vi "UHR-Fleezers Control (fpga) - 11.7.1UCBMeng3RG1.vi"() -> ()   [LabVIEW 2014]
doc: "UHR-Fleezers Instrument Control Code (fpga)"
uses:
  <vilib>/Platform/TimedLoop/XDataNode/timing_clust.ctl
  <vilib>/Platform/TimedLoop/XDataNode/nitl_modes.ctl
  <vilib>/Platform/TimedLoop/XDataNode/wakeup.ctl
  <vilib>/rvi/Emulation/niFpgaGetClockAttributes.vi
  <vilib>/rvi/Emulation/niFpgaSctlEmulationGetInTimedLoop.vi
  <vilib>/rvi/Emulation/niFpgaEmulationReportErrorSimple.vi
  <vilib>/rvi/Emulation/niFpgaProcessEmulError.vi
  <vilib>/rvi/DataTransferAndStorage/Container/Common/niFpgaContainerExecOnDevCompGetState.vi
  <vilib>/rvi/Emulation/niFpgaEmulationIsFPGAContextNoSignature.vi
  <vilib>/rvi/DataTransferAndStorage/Container/Common/niFpgaContainerGetUniqueNameForEmu.vi
  <vilib>/rvi/errors/nirviReportUnexpectedCaseInternalError (U32).vi
  <vilib>/rvi/Memory/Memory_Emulation/niFpgaMemoryEmulationCacheClearOnFirstRun.vi
  <vilib>/rvi/Memory/Memory_Emulation/nirvimemoryEmulationManagerCache_MakeExclusive.vi
  <vilib>/rvi/Memory/Memory_Emulation/niFpgaMemoryEmulationValidateCache.vi
  <vilib>/rvi/Memory/Memory_Emulation/nirvimemoryEmulationManagerCache_InsertValue.vi
  <vilib>/Utility/error.llb/Clear Errors.vi
  <vilib>/rvi/Memory/Memory_Emulation/nirvimemoryEmulationManagerCache_ReleaseExclusive.vi
  <vilib>/rvi/Memory/Memory_Emulation/nirvimemoryEmulationManagerCache_GetValue.vi
  <vilib>/rvi/Memory/Memory_Emulation/nirvimemoryEmulationManagerCache_SetValue.vi
  <vilib>/rvi/Emulation/niFpgaSctlEmulationResourceMgr.vi
  <vilib>/rvi/Emulation/niFpgaCriticalErrorInLSC.vi
  <vilib>/rvi/eio/common/nirviEmuTemplateMethod_errors.vi
  <vilib>/rvi/interface/RandomDataEmulation/niFpgaRandomDataHandleErrors.vi
  <vilib>/rvi/DataTransferAndStorage/Container/XNode/niFpgaContainer.xnode
  <vilib>/rvi/Memory/Memory_Emulation/niFpgaMemoryEmulationRefIn.vi
  <vilib>/eio/EIONode/EIONode.xnode
  <vilib>/eio/EIOMethodNode/EIOMethodNode.xnode
  <vilib>/rvi/interface/RandomDataEmulation/nirviRandomDataFpgaReadWriteTemplate.vi
  <vilib>/addons/control/pid/fpga.llb/XNode/niFpgaPID.xnode
  <vilib>/Platform/TimedLoop/XDataNode/XDataNode.xnode
  <vilib>/Platform/TimedLoop/XDataNode/XDNodeRunTimeDep.lvlib
panel:
  in  "Address 2":u32
  in  "Data":i64
  in  "Ready Write":bool
  in  "Tab Control":T1(tab)=enum."Force FB"
  in  "Set 3":bool
  in  "Set 2":bool=TRUE
  in  "Set 1":bool=TRUE
  in  "Trap Pos to FIFO":bool
  in  "N of AI1 Int Acq Sets":i16=2 min=1 max=3 step=1
  out "AI Late Counter":u8
  in  "ai count":u16=400
  in  "+ phase":bool
  in  "Phase count adjustment":i16
  out "Relative phase":i16
  in  "AI to FIFO":bool
  out "BD1 Frequency Out 1":u64
  out "BD1 Frequency Out 2":u64
  out "Trap Pos FIFO Timeout":u16
  out "Trap AI FIFO Timeout":u16
  in  "Trap FIFO Set Timeout":i32
  in  "Tab Control 2":T2(tab)
  in  "RD":bool
  in  "FB1 output high":i16=3000
  in  "FB1 output low":i16
  in  "D1":i16
  in  "I1":i16=5
  in  "P1":i16=10
  in  "Swap F1 and F2":bool
  in  "Cont. Scan":bool
  in  "Abort scan":bool
  in  "Cycles per step":u64
  in  "Scan BD":bool
  in  "Number of scans":u16
  in  "Scan steps":u64
  in  "Scan freq.  increment":i64
  out "Scanning":bool
  in  "Start scan":bool
  in  "OSK Bd 1":bool
  in  "Reset Bd 1":bool
  in  "PMODE":bool
  in  "Direct RF Box \nCommunication":bool
  in  "Data BD 2":u8 format="%08b"
  in  "Data BD 1":u8 format="%08b"
  in  "Address":u8 format="%02x"
  in  "Update Data":bool
  in  "FPGA Controls\n RF Box":bool
  in  "Number Interlace Cycles":u8=2 min=1 max=3
  in  "Interlace Off Parameters":u8=1 min=1 max=3
  in  "Interlace ON/OFF":bool
  out "DIO Relative phase":i16
  in  "Phase count adjustment (DIO)":i16
  in  "+ phase (DIO)":bool
  out "DIO Late Counter":u8
  in  "DIO count 1 (ticks)":u16=400
  in  "DIO count 2 (ticks)":u16=400
  in  "DIO count 3 (ticks)":u16=400
  out "AI2 Y Sum Set 2":i16
  out "AI2 Y Sum Set 1":i16
  in  "FB Setpoint Set 1":i16 min=0 step=1
  in  "FB Reset Set 1":bool
  in  "FB On/Off Set 1":bool
  in  "FB Reset Set 2":bool
  in  "FB On/Off Set 2":bool
  in  "FB Setpoint Set 2":i16 min=0 step=1
  out "Scan I":u64
  in  "Amp switch delay":u8=5
  in  "XY phase ext loop method":bool
  in  "BD 2 Amplitude 1":u16
  in  "BD 1 Amplitude 1":u16
  in  "BD 2 Frequency 1":u64
  in  "BD 1 Frequency 1":u64
  in  "BD 2 Amplitude 2":u16
  in  "BD 1 Amplitude 2":u16
  in  "BD 2 Frequency 2":u64
  in  "BD 1 Frequency 2":u64
  in  "BD 2 Amplitude 3":u16
  in  "BD 1 Amplitude 3":u16
  in  "BD 2 Frequency 3":u64
  in  "BD 1 Frequency 3":u64
  in  "BD 1 Delay (ticks)":u8
  in  "BD 2 Delay (Ticks)":u8 caption="Count(Ticks)"
  in  "Next trap write delay (ticks)":u8 caption="Count(Ticks)"
  in  "Trap 1 osc enable":bool
  in  "Trap 2 osc enable":bool
  in  "FB2 output high":fxp<+/-,16,1>=0.999969482421875
  in  "FB2 output low":fxp<+/-,16,1>=-1.0
  in  "P2":fxp<+/-,16,8> format="%.11g"
  in  "I2":fxp<+/-,16,8>=10.0 format="%.11g"
  in  "D2":fxp<+/-,16,8> format="%.11g"
  in  "Negate Diff?":bool
  in  "Diff FB Measurement?":bool
  in  "FB Trig Integrate":u32=1
  out "TTrig?":bool
  in  "TTrig Negate Pos":bool=TRUE
  out "Trap Pos FB Int Signal":fxp<+/-,24,9> format="%.18g"
  out "Trap Pos FB Int-Norm Signal":fxp<+/-,16,1> format="%.16g"
  in  "FPGA TTrig Thresh":i64
  in  "FPGA Trap Trig":bool
  out "Trap Pos FB Action":i64
  in  "Trap Pos. FB Offset Factor":i64
  in  "Trap Pos. FB Mult Factor":i64=2
  in  "Trap Pos. FB Reset":bool
  in  "Trap Pos FB Monitor T1 or T2":bool
  in  "AI1 X Scale":u16
  in  "Trap Pos FB Int Count":u16=100
  in  "Trap Pos FB Negate Action":bool
  out "AI1 X Set 2":fxp<+/-,16,1>
  out "AI1 X Set 1":fxp<+/-,16,1>
  in  "Trap Pos. FB SP":fxp<+/-,16,1>
  in  "Force feedback":bool
  out "TTrig Sig":i64
  out "TTrig Fin Thresh":i64
  in  "1D or 2D Scan?":bool
  in  "Abort scan (MCL)":bool
  in  "MCL Scan Axis":bool
  in  "Cont. Scan (MCL)":bool
  out "Scan I (MCL)":u64
  in  "Number of scans (MCL)":u16
  out "Scanning MCL":bool
  in  "Scan steps (MCL)":u64
  in  "Cycles per step (MCL)":u64
  in  "Scan freq.  increment (MCL)":i16
  in  "Start scan (MCL)":bool
  in  "AO2":i16
  in  "AO1":i16
  out "MCL Late Counter":u8
  in  "MCL count":u32=800
  out "MCL Relative Phase":i16
  in  "Phase count adjustment (MCL)":i16
  in  "+ phase (MCL)":bool
  out "APD2 int gate":bool
  out "APD3 out state":bool
  in  "APD Gate Operating Mode":u8 max=2 step=1
  in  "Invert APD Gate":bool
  in  "APD Gate OFF Count":u16=100
  in  "APD Gate ON Count":u16=300
  out "APD 1 Gate Late Counter":u8
  out "APD 1 Gate Relative Phase":i16
  in  "Phase count adjustment (APD 1 Gate)":i16
  in  "+ phase (APD 1 Gate)":bool
  out "APD 2 Counts 0":u32
  out "APD 2 Counts 1":u32
  out "APD 1 Counts 0":u32
  out "APD 1 Counts 1":u32
  out "APD1 out state":bool
  in  "APD AO scale factor":i16=1
  in  "APD to FIFO":bool
  in  "APD Acq Rate Count":u32=20000000
  out "APD Acq Late Counter":u8
  out "APD Acq Relative Phase":i16
  in  "Phase Count Adjustment (APD Acq)":i16
  in  "+ phase (APD Acq)":bool
  in  "Phase count adjustment (APD 2 Gate)":i16
  out "APD 2 Gate Late Counter":u8
  out "APD 2 Gate Relative Phase":i16
  in  "+ phase (APD 2 Gate)":bool
  out "APD2 out state":bool
  out "APD 3 Counts 0":u32
  out "APD 3 Counts 1":u32
  out "APD 3 Gate Late Counter":u8
  in  "Phase count adjustment (APD 3 Gate)":i16
  out "APD 3 Gate Relative Phase":i16
  in  "+ phase (APD 3 Gate)":bool
  out "APD1 int gate":bool
  out "APD3 int gate":bool
  in  "D3":i16
  in  "I3":i16=5
  in  "P3":i16=10
  in  "Green Filter Flipper":bool
  in  "Green FB Count":u16=1200
  out "Green Late Counter":u8
  out "Green FB Relative Phase":i16
  in  "Phase count adjustment (Green FB)":i16=10
  in  "+ phase (Green FB)":bool
  out "Green FB Sum":i16
  in  "Green int current ON count adj":u16=150
  in  "Current Out":u16=30000
  in  "Green FB On/Off":bool
  in  "Green FB Setpoint":i16=250 min=0 step=1
  in  "Green FB Reset":bool
  in  "Operating Mode 2":u8=2 max=2 step=1
  in  "Invert GI 2":bool
  in  "Green interlace OFF count 2":u16=900
  in  "Green interlace ON count 2":u16=300
  out "GI Late Counter 2":u8
  out "GI Relative phase 2":i16
  in  "Phase count adjustment (GI) 2":i16=20
  in  "+ phase (GI) 2":bool
  in  "Green interlace OFF count":u16=100
  out "GI Relative phase":i16
  in  "Phase count adjustment (GI)":i16
  in  "+ phase (GI)":bool
  in  "Green interlace ON count":u16=300
  out "GI Late Counter":u8
  in  "Invert GI":bool
  in  "Operating Mode":u8 max=2 step=1
  in  "+ phase (RI)":bool
  out "RI Relative phase":i16
  out "RI Late Counter":u8
  in  "Red interlace ON count":u16=300
  in  "Red interlace OFF count":u16=100
  in  "Invert RI":bool
  in  "Red Laser Operating Mode":u8 max=2 step=1
  in  "Phase count adjustment (RI)":i16
  out "Red FB Intensity":i16
  in  "RI Current Out":u16=30000
  in  "Red FB On/Off":bool
  in  "D4":i16
  in  "I4":i16=5
  in  "P4":i16=10
  in  "Red FB Setpoint":i16=250 min=0 step=1
  in  "Red FB Reset":bool
  in  "RI Operating Mode 2":u8=2 max=2 step=1
  in  "Invert RI 2":bool
  in  "Phase count adjustment (BI AO)":i16=20
  in  "Blue current ON count adj (AO)":u16=150
  in  "BI Current Out":i16=30000
  in  "Blue FB On/Off":bool
  in  "D5":i16
  in  "I5":i16=5
  in  "P5":i16=10
  in  "Blue FB Setpoint":i16=250 min=0 step=1
  in  "Blue FB Reset":bool
  in  "BI Operating Mode (AO)":u8=2 max=2 step=1
  in  "Invert BI (AO)":bool
  in  "Blue OFF count (AO)":u16=900
  in  "Blue ON count (AO)":u16=300
  out "BI Late Counter (AO)":u8
  out "BI Relative phase (AO)":i16
  in  "+ phase (BI AO)":bool
  in  "Phase count adjustment (BI D)":i16
  in  "Blue Laser Operating Mode (D)":u8 max=2 step=1
  in  "Invert BI (D)":bool
  in  "Blue interlace OFF count (D)":u16=100
  in  "Blue interlace ON count (D)":u16=300
  out "Blue Late Counter (D)":u8
  out "BI Relative phase (D)":i16
  in  "+ phase (BI D)":bool
  out "Blue Intensity":i16
  # "Only one of these can be on\nat a time:"
  # "Raster Scan AOD"
  # "1 (X)"
  # "2 (Y)"
  # "IR Intensity Feedback (RF BD 1)"
  # "FB Gains Set 1"
  # "FB output range 1"
  # "False is usual, True is external loop method"
  # "Parameters if using the external RF switching loop"
  # "Parameters if using the usual internal RF switching method"
  # "FB Triggering Excitation Laser"
  # "Trap Pos. FB Gains"
  # "Trap Pos. FB Range"
  # "AO1 (Y)"
  # "2D"
  # "1D"
  # "AO2 (X)"
  # "APD AO for aligning"
  # "Detection Loop"
  # "Green fluorescent laser digital gate interlacing loop"
  # "0 Forced ON\n1 Forced OFF\n2 Interlacing"
  # "Green FB Gains"
  # "Red fluorescent laser digital gate interlacing loop"
  # "Detection Loop"
  # "0 Forced ON\n1 Forced OFF\n2 Interlacing"
  # "Analog/FB Control Loop\n(Disabled)"
  # "Digital Control Loop"
  # "Blue laser intensity reading"
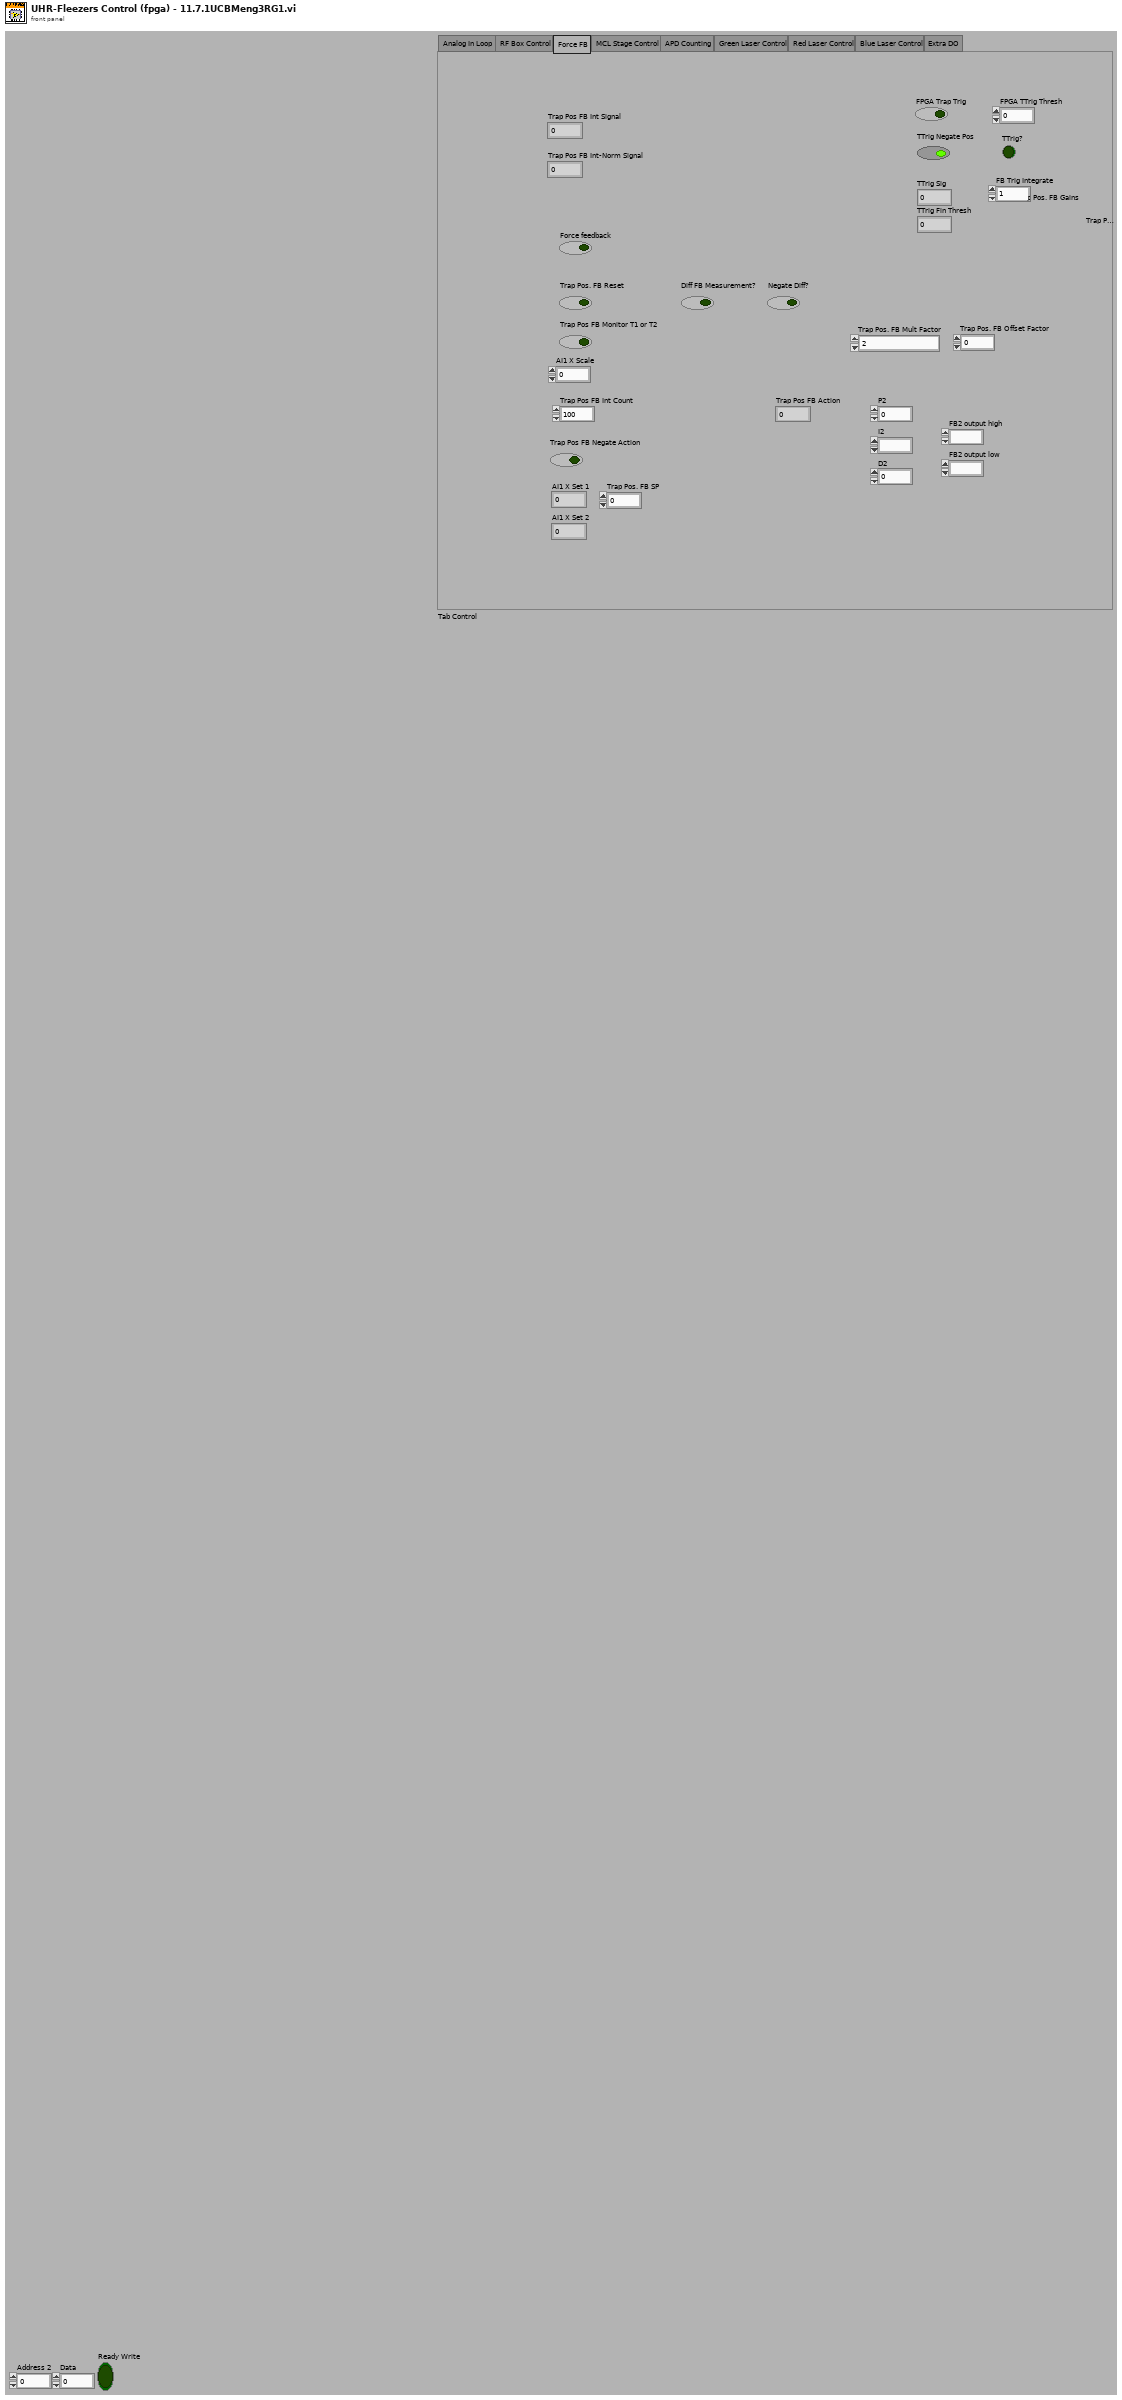
[diagram p1: front panel]
types:
  T1 = enum32{"Analog In Loop", "RF Box Control", "Force FB", "MCL Stage Control", "APD Counting", "Green Laser Control", "Red Laser Control", "Blue Laser Control", "Extra DO"}
  T2 = enum32{"Controls", "Interlacing Frequency and Amplitude Values", "Oscillate trap from memory"}
  T3 = typedef "XDNodeRunTimeDep.lvlib/timing_clust.ctl" = cluster{"Expected End [f-1]":u64, "Actual End [f-1]":u64, "Finished Late? [f-1]":bool, "Expected End [i-1]":u64, "Actual End [i-1]":u64, "Finished Late? [i-1]":bool, "Expected Start [i]":u64, "Actual Start [i]":u64, "Expected Start [f]":u64, "Actual Start [f]":u64, "Source Name":string, "Structure Name":string, "Period":i64, "Deadline":i64, "Offset":i64, "Start":i64, "Priority":i32, "Timeout":i32, "Mode":T4, "Wakeup Reason":T5, "Error":errorcluster, "Source Type":string, "Secondary Source Type":string, "Global End Time":u64, "Global Start Time":u64, "Frame Duration":u64, "Iteration Duration":u64, "Assigned CPU":i32, "I/O Scan Engine Mode":u32}
  T4 = typedef "XDNodeRunTimeDep.lvlib/nitl_modes.ctl" = enum32{"No Change", "Process missed periods, maintain original phase", "Discard missed periods, maintain original phase", "Process missed periods, ignore original phase", "Discard missed periods, ignore original phase"}
  T5 = typedef "XDNodeRunTimeDep.lvlib/wakeup.ctl" = enum32{"Normal", "Aborted", "Asynchronous wakeup", "Timing source error", "Timed loop error", "Timeout"}
  T6 = cluster{"proportional gain (Kc)":i16, "integral gain (Kc*Ts/Ti)":i16, "derivative gain (Kc*Td/Ts)":i16}
  T7 = cluster{"FB1 output high":i16, "FB1 output low":i16}
  T8 = cluster{"P2":fxp<+/-,16,8>, "I2":fxp<+/-,16,8>, "D2":fxp<+/-,16,8>}
  T9 = cluster{"FB2 output high":fxp<+/-,16,1>, "FB2 output low":fxp<+/-,16,1>}
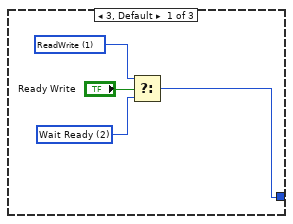
[diagram p2: hidden frame]
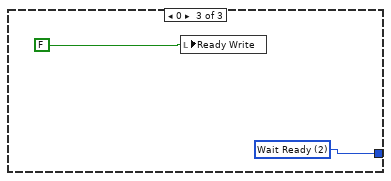
[diagram p3: hidden frame]
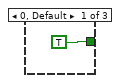
[diagram p5: hidden frame]
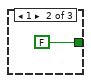
[diagram p6: hidden frame]
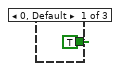
[diagram p7: hidden frame]
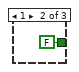
[diagram p8: hidden frame]
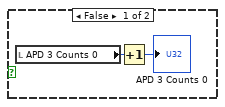
[diagram p10: hidden frame]
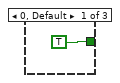
[diagram p11: hidden frame]
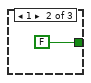
[diagram p12: hidden frame]
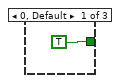
[diagram p13: hidden frame]
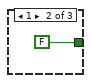
[diagram p14: hidden frame]
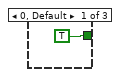
[diagram p15: hidden frame]
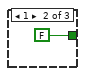
[diagram p16: hidden frame]
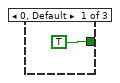
[diagram p17: hidden frame]
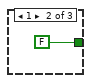
[diagram p18: hidden frame]
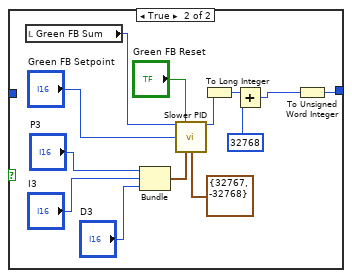
[diagram p20: hidden frame]
diagram:
  w1 = i16 2 items=["UnSet Ready", "ReadWrite", "Wait Ready"]
  w4 = u16 0
  w6 = FALSE
  w3 = FALSE
  # "timing array current index"
  # "timing array"
  # "timing counter (phase adjusted here)"
  # "late counter"
  n1 = flat-sequence "FPGA initialization to do before running any of the loops" {
    tunnel: [u16 0 ("DIO count 3 (ticks)")] -> w2
    tunnel: [w14] -> _
    frame #0 {
      w13 = FALSE ("Enable")
      # "BD 2 (Y)"
      # "BD 1 (X)"
      # "Start up expansion chassis early\nto avoid delays later"
      # "This pin controls udclk on the RF boards.\nWhen initially configuring the boards, this pin needs to be\nconfigured as a high impedance input.  Later it will be switched\nto an output."
      # "Initial setting of DIO data and \naddress to low (before reset).  \nThis needs to happen before the other\ncontrol method loops execute."
      n2 = xnode "FPGA I/O Node"("Chassis2/Mod1/AO0"=u16 0 ("Chassis2/Mod4/AO0")) -> ("Chassis2/Mod2/AI0"=w14:i16)  [unwired: 2 in, 2 out]
      n3 = xnode "FPGA I/O Method Node"("Enable"=w13) -> ()  [unwired: 1 in, 1 out]
      n4 = xnode "FPGA I/O Method Node"("Enable"=w13) -> ()  [unwired: 1 in, 1 out]
      n5 = xnode "FPGA I/O Node"("Connector1/DIO0"=FALSE, "Connector1/DIO1"=FALSE, "Connector1/DIO2"=FALSE, "Connector1/DIO3"=FALSE, "Connector1/DIO4"=FALSE, "Connector1/DIO5"=FALSE, "Connector1/DIO6"=FALSE, "Connector1/DIO7"=FALSE, "Connector1/DIO8"=FALSE, "Connector1/DIO9"=FALSE, "Connector1/DIO10"=FALSE, "Connector1/DIO11"=FALSE, "Connector1/DIO12"=FALSE, "Connector1/DIO13"=FALSE, "Connector1/DIO15"=FALSE, "Connector1/DIO20"=FALSE, "Connector1/DIO21"=FALSE, "Connector1/DIO22"=FALSE, "Connector1/DIO23"=FALSE, "Connector1/DIO24"=FALSE, "Connector1/DIO25"=FALSE, "Connector1/DIO26"=FALSE, "Connector1/DIO27"=FALSE, "Connector1/DIO14"=FALSE) -> ()  [unwired: 24 in, 24 out]
    }
  }
  n6 = local read "AO1"() -> (w11:i16)
  n7 = local read "AO2"() -> (w10:i16)
  n8 = node-c288() -> (w9:T3)  [unwired: 1 in]
  n9 = To Unsigned Long Integer(number=w2) -> (unsigned 32bit integer=w7:u32)
  n10 = timed-loop "RF box board DIO control: control bits" {
    timing: w9 -> [_]
    timing-out: [_] -> w8
    tunnel: [w43] -> _
    tunnel: w2 -> [w43]
    stop <- FALSE stop-if-true
    n11 = xnode "FPGA I/O Node"("Connector1/DIO16"="RD", "Connector1/DIO17"="PMODE", "Connector1/DIO18"="OSK Bd 1", "Connector1/DIO19"="Reset Bd 1", "Connector0/DIO3"="Green Filter Flipper") -> ()  [unwired: 5 in, 5 out]
  }
  n12 = while "RF box board direct communication loop" {
    tunnel: w2 -> [_]
    stop <- FALSE stop-if-true
    n13 = case "Whether to use direct communication method (only use one method at a time)" shown="True" "Direct RF Box \nCommunication" {
      frame False {
      }
      frame True {
        n14 = case shown="True" "Update Data" {
          frame False {
          }
          frame True {
            n15 = flat-sequence {
              frame #0 {
                n16 = First Call?() -> (First Call?: T/F=w53:bool)
                n17 = case shown="True" w53 {
                  frame False {
                  }
                  frame True {
                    # "If first time data updated, be sure to set WR high\nbefore setting data and address bits."
                    n18 = flat-sequence {
                      frame #0 {
                        n19 = xnode "FPGA I/O Node"("Connector1/DIO15"=TRUE) -> ()  [unwired: 1 in, 1 out]
                      }
                      frame #1 {
                        n20 = call "Wait"("Count(Ticks)"=u8 40 ("DO Delay 3 (Ticks)")) -> ()  [unwired: 1 out]
                      }
                    }
                  }
                }
              }
              frame #1 {
                n21 = Number To Boolean Array(number="Address") -> (Boolean array=w102:bool[])
                n22 = Number To Boolean Array(number="Data BD 1") -> (Boolean array=w103:bool[])
                n23 = Number To Boolean Array(number="Data BD 2") -> (Boolean array=w72:bool[])
                n24 = Index Array(array=w103, index=7) -> (element=w87:bool)
                n25 = Index Array(array=w103, index=6) -> (element=w86:bool)
                n26 = Index Array(array=w103, index=5) -> (element=w85:bool)
                n27 = Index Array(array=w103, index=4) -> (element=w84:bool)
                n28 = Index Array(array=w103, index=3) -> (element=w83:bool)
                n29 = Index Array(array=w103, index=2) -> (element=w82:bool)
                n30 = Index Array(array=w103, index=1) -> (element=w81:bool)
                n31 = Index Array(array=w103, index=0) -> (element=w80:bool)
                n32 = Index Array(array=w102, index=5) -> (element=w79:bool)
                n33 = Index Array(array=w102, index=4) -> (element=w78:bool)
                n34 = Index Array(array=w102, index=3) -> (element=w77:bool)
                n35 = Index Array(array=w102, index=2) -> (element=w76:bool)
                n36 = Index Array(array=w102, index=1) -> (element=w75:bool)
                n37 = Index Array(array=w102, index=0) -> (element=w74:bool)
                n38 = Index Array(array=w72, index=7) -> (element=w63:bool)
                n39 = Index Array(array=w72, index=6) -> (element=w62:bool)
                n40 = Index Array(array=w72, index=5) -> (element=w61:bool)
                n41 = Index Array(array=w72, index=4) -> (element=w60:bool)
                n42 = Index Array(array=w72, index=3) -> (element=w59:bool)
                n43 = Index Array(array=w72, index=2) -> (element=w58:bool)
                n44 = Index Array(array=w72, index=1) -> (element=w57:bool)
                n45 = Index Array(array=w72, index=0) -> (element=w56:bool)
                n46 = xnode "FPGA I/O Node"("Connector1/DIO0"=w87, "Connector1/DIO1"=w86, "Connector1/DIO2"=w85, "Connector1/DIO3"=w84, "Connector1/DIO4"=w83, "Connector1/DIO5"=w82, "Connector1/DIO6"=w81, "Connector1/DIO7"=w80, "Connector1/DIO8"=w79, "Connector1/DIO9"=w78, "Connector1/DIO10"=w77, "Connector1/DIO11"=w76, "Connector1/DIO12"=w75, "Connector1/DIO13"=w74, "Connector1/DIO20"=w63, "Connector1/DIO21"=w62, "Connector1/DIO22"=w61, "Connector1/DIO23"=w60, "Connector1/DIO24"=w59, "Connector1/DIO25"=w58, "Connector1/DIO26"=w57, "Connector1/DIO27"=w56) -> ()  [unwired: 22 in, 22 out]
              }
              frame #2 {
                # "wait and then apply write signal"
                n47 = call "Wait2"("Count(Ticks)"=u8 40 ("DO Delay 1 (Ticks)")) -> ()  [unwired: 1 out]
              }
              frame #3 {
                # "sending bit low writes data to board buffer"
                n48 = xnode "FPGA I/O Node"("Connector1/DIO15"=FALSE) -> ()  [unwired: 1 in, 1 out]
              }
              frame #4 {
                # "wait then return write signal"
                n49 = call "Wait3"("Count(Ticks)"=u8 40 ("DO Delay 2 (Ticks)")) -> ()  [unwired: 1 out]
              }
              frame #5 {
                # "sending bit high makes ready to\nwrite more data"
                n50 = xnode "FPGA I/O Node"("Connector1/DIO15"=TRUE) -> ()  [unwired: 1 in, 1 out]
              }
            }
          }
        }
      }
    }
  }
  n51 = while "RF box board DIO control: parallel communication" {
    shift-right: [w116] -> _
    shift-left: w2 -> [w115]
    shift-right: [w114] -> _
    shift-left: FALSE ("Swap F1 and F2") -> [w113]
    stop <- FALSE stop-if-true
    n52 = flat-sequence {
      tunnel: w113 -> [w120]
      tunnel: w115 -> [w118]
      tunnel: [w120] -> w112
      tunnel: [w119] -> w111
      tunnel: [w118] -> w110
      tunnel: [w126] -> w116
      tunnel: [w125] -> w114
      tunnel: w112 -> [w124]
      tunnel: w111 -> [w122]
      tunnel: w110 -> [w121]
      frame #0 {
        n53 = call "Loop Timer"("Count(Ticks)"=w118) -> ("Tick Count(Ticks)"=w119:u16)
      }
      frame #1 {
        n54 = flat-sequence {
          tunnel: ["FPGA Controls\n RF Box"] -> w123
          tunnel: w124 -> [w127]
          tunnel: [w180] -> w126
          tunnel: [w193] -> w125
          tunnel: w123 -> [w192]
          tunnel: w122 -> [w186]
          tunnel: w121 -> [w183]
          frame #0 {
            n55 = case shown="True" "FPGA Controls\n RF Box" {
              tunnel: w127 -> [_ w129]
              frame False {
              }
              frame True {
                n56 = flat-sequence {
                  tunnel: w129 -> [w139]
                  frame #0 {
                    n57 = First Call?() -> (First Call?: T/F=w130:bool)
                    n58 = case shown="True" w130 {
                      frame False {
                      }
                      frame True {
                        # "BD 2"
                        # "BD 1"
                        # "If first time data updated, be sure to set WR high and UDCLK low\nbefore setting data and address bits."
                        n59 = xnode "FPGA I/O Method Node"("Enable"=TRUE) -> ("FPGA I/O Out"=w132:refnum<k21>)  [unwired: 1 in]
                        n60 = xnode "FPGA I/O Method Node"("Enable"=TRUE) -> ("FPGA I/O Out"=w135:refnum<k21>)  [unwired: 1 in]
                        n61 = xnode "FPGA I/O Node"("Connector1/DIO15"=TRUE) -> ()  [unwired: 1 in, 1 out]
                        n62 = xnode "FPGA I/O Node"("I/O Item"=FALSE ("Connector1/DIO30"), "FPGA I/O In"=w132) -> ()  [unwired: 1 out]
                        n63 = xnode "FPGA I/O Node"("I/O Item"=FALSE ("Connector1/DIO30"), "FPGA I/O In"=w135) -> ()  [unwired: 1 out]
                      }
                    }
                  }
                  frame #1 {
                    n64 = case shown="False" FALSE {
                      tunnel: w139 -> [w141 _]
                      frame False {
                        # "Usual operation"
                        n65 = flat-sequence "BD 1 (X)" {
                          tunnel: w141 -> [w148]
                          tunnel: "Amp switch delay" -> [w149]
                          frame #0 {
                            n66 = call "Wait6"("Count(Ticks)"="BD 1 Delay (ticks)") -> ()  [unwired: 1 out]
                          }
                          frame #1 {
                            # "switch frequency"
                            n67 = xnode "FPGA I/O Node"("Connector1/DIO36"=w148) -> ()  [unwired: 1 in, 1 out]
                          }
                          frame #2 {
                            # "~5 ticks is usual"
                            n68 = call "Wait4"("Count(Ticks)"=w149) -> ()  [unwired: 1 out]
                          }
                          frame #3 {
                            # "this switches amplitude"
                            # "switch amplitude"
                            # "send udclk high"
                            n69 = xnode "FPGA I/O Node"("Connector1/DIO30"=TRUE ("Connector1/DIO15")) -> ()  [unwired: 1 in, 1 out]
                          }
                          frame #4 {
                            # "reset to be ready for next\ncycle"
                            # "send udclk low"
                            n70 = xnode "FPGA I/O Node"("Connector1/DIO30"=FALSE ("Connector1/DIO15")) -> ()  [unwired: 1 in, 1 out]
                          }
                        }
                        n71 = flat-sequence "BD 2 (Y)" {
                          tunnel: w141 -> [w143]
                          tunnel: "Amp switch delay" -> [w144]
                          frame #0 {
                            n72 = call "Wait7"("Count(Ticks)"="BD 2 Delay (Ticks)") -> ()  [unwired: 1 out]
                          }
                          frame #1 {
                            # "switch frequency"
                            n73 = xnode "FPGA I/O Node"("Connector1/DIO37"=w143) -> ()  [unwired: 1 in, 1 out]
                          }
                          frame #2 {
                            # "~5 ticks is usual"
                            n74 = call "Wait5"("Count(Ticks)"=w144) -> ()  [unwired: 1 out]
                          }
                          frame #3 {
                            # "this switches amplitude"
                            # "switch amplitude"
                            # "send udclk high"
                            n75 = xnode "FPGA I/O Node"("Connector1/DIO29"=TRUE ("Connector1/DIO15")) -> ()  [unwired: 1 in, 1 out]
                          }
                          frame #4 {
                            # "reset to be ready for next\ncycle"
                            # "send udclk low"
                            n76 = xnode "FPGA I/O Node"("Connector1/DIO29"=FALSE ("Connector1/DIO15")) -> ()  [unwired: 1 in, 1 out]
                          }
                        }
                      }
                      frame True {
                        # "Operation when you need a long delay for either X or Y to synchonize AOD light out phase (> ~100 ticks)."
                        # "Trigger the external loop by sending the boolean FSK value through a FIFO"
                      }
                    }
                  }
                }
              }
            }
          }
          frame #1 {
            # "This is the prior cycle's on time"
            # "increment timing\nindex, reset to 0 if \nend of matrix"
            # "Reset to begginning (1) when number of cycles reached."
            # "timing index"
            # "build byte stacks for writing data\n(must correspond to addresses array constant)"
            # "Timing housekeeping"
            # "Adjust phase if late\n(maintains constant phase relationship between cycles)"
            n77 = Bundle("FB1 output high"="FB1 output high", "FB1 output low"="FB1 output low") -> (w153:T7)  [unwired: 1 in]
            n78 = Bundle("P1"="P1", "I1"="I1", "D1"="D1") -> (w154:cluster{"P1":i16, "I1":i16, "D1":i16})  [unwired: 1 in]
            n79 = feedback #1(u8 0 ("t")) -> (w189:u8)
            n80 = Increment(x=w189) -> (x+1=w232:u8)
            n81 = Increment(x="Number Interlace Cycles") -> (x+1=w227:u8)
            n82 = Equal?(x=w232, y=w227) -> (x = y?=w234:bool)
            n83 = Select(t=u8 1, s=w234, f=w232) -> (s? t:f=w188:u8)
            n84 = feedback-in #1(w188) -> ()
            n85 = Increment(x=w188) -> (x+1=w229:u8)
            n86 = Equal?(x=w229, y=w227) -> (x = y?=w230:bool)
            n87 = Select(t=u8 1, s=w230, f=w229) -> (s? t:f=w226:u8)
            n88 = Select(t=w226, s="Interlace ON/OFF", f="Interlace Off Parameters") -> (s? t:f=w152:u8)
            n89 = case shown="2" w152 {
              tunnel: [w312 w468 "BD 1 Frequency 3"] -> w222
              tunnel: [w311 "BD 2 Frequency 2" "BD 2 Frequency 3"] -> w211
              tunnel: ["BD 2 Amplitude 1" "BD 2 Amplitude 2" "BD 2 Amplitude 3"] -> w168
              tunnel: [w300 w473 "BD 1 Amplitude 3"] -> w171
              tunnel: w154 -> [w274 w470 _]
              tunnel: w153 -> [w275 w469 _]
              frame 1, Default {
                w291 = fxp<+/-,24,9> 0.0 ("AI1 X Set 2")
                w284 = u16 0
                w307 = u64 0 ("f")
                # "This signal integration happens no matter what\nso that correct setpoints can be chosen before \nturning on the FB."
                # "Trap 1"
                n90 = local read "AI1 X Set 2"() -> (w287:fxp<+/-,16,1>)
                n91 = local read "AI1 X Set 1"() -> (w288:fxp<+/-,16,1>)
                n92 = local read "Scanning"() -> (w313:bool)
                n93 = Or(x=w313, y="Start scan") -> (x .or. y?=w305:bool)
                n94 = case shown="False" "Diff FB Measurement?" {
                  tunnel: w287 -> [w321 w330]
                  tunnel: w288 -> [w320 w331]
                  tunnel: [w318 w322] -> w289
                  frame False {
                    n95 = Select(t=w320, s="Trap Pos FB Monitor T1 or T2", f=w321) -> (s? t:f=w318:fxp<+/-,16,1>)
                  }
                  frame True {
                    n96 = Subtract(x=w331, y=w330) -> (x-y=w323:fxp<+/-,17,2>)
                    n97 = Not(x="Negate Diff?") -> (.not. x?=w329:bool)
                    n98 = Boolean To (0,1)(Boolean="Negate Diff?") -> (0, 1=w327:i16)
                    n99 = Boolean To (0,1)(Boolean=w329) -> (0, 1=w328:i16)
                    n100 = Negate(x=w327) -> (-x=w326:i16)
                    n101 = Add(x=w326, y=w328) -> (x+y=w324:i16)
                    n102 = Multiply(x=w324, y=w323) -> (x*y=w322:fxp<+/-,32,17>)
                  }
                }
                n103 = Not(x="Abort scan") -> (.not. x?=w303:bool)
                n104 = And(x=w303, y=w305) -> (x .and. y?=w302:bool)
                n105 = case "For raster scanning" shown="True" w302 {
                  tunnel: [u64 0 w457] -> w308
                  tunnel: "Start scan" -> [_ w442]
                  frame False {
                    n106 = local write "Scanning"(FALSE ("scanning")) -> ()
                  }
                  frame True {
                    w426 = i64 0
                    w425 = u64 0
                    # "scan incr."
                    # "freq. incr. mult."
                    # "count steps"
                    # "count number of cycles"
                    n107 = feedback #2(w425) -> (w454:u64)
                    n108 = Select(t=w425, s=w442, f=w454) -> (s? t:f=w456:u64)
                    n109 = Increment(x=w456) -> (x+1=w453:u64)
                    n110 = Greater?(x="Cycles per step", y=w453) -> (0:w435:bool)
                    n111 = Select(t=w453, s=w435, f=w425) -> (s? t:f=w452:u64)
                    n112 = feedback-in #2(w452) -> ()
                    n113 = feedback #3(w425) -> (w451:u64)
                    n114 = Select(t=w425, s=w442, f=w451) -> (s? t:f=w446:u64)
                    n115 = Increment(x=w446) -> (x+1=w450:u64)
                    n116 = Add(x="Scan steps", y="Scan steps") -> (x+y=w449:u64)
                    n117 = Select(t=w446, s=w435, f=w450) -> (s? t:f=w430:u64)
                    n118 = Greater?(x=w449, y=w430) -> (0:w429:bool)
                    n119 = Select(t=w430, s=w429, f=w425) -> (s? t:f=w447:u64)
                    n120 = feedback-in #3(w447) -> ()
                    n121 = Equal?(x="Scan steps", y=w430) -> (x = y?=w434:bool)
                    n122 = Greater?(x="Scan steps", y=w446) -> (0:w445:bool)
                    n123 = feedback #4(w426) -> (w448:i64)
                    n124 = Select(t=w426, s=w442, f=w448) -> (s? t:f=w432:i64)
                    n125 = Increment(x=w432) -> (x+1=w444:i64)
                    n126 = Decrement(x=w432) -> (x-1=w443:i64)
                    n127 = Select(t=w444, s=w445, f=w443) -> (s? t:f=w433:i64)
                    n128 = Select(t=w432, s=w434, f=w433) -> (s? t:f=w431:i64)
                    n129 = Select(t=w432, s=w435, f=w431) -> (s? t:f=w427:i64)
                    n130 = Select(t=w427, s=w429, f=w426) -> (s? t:f=w428:i64)
                    n131 = feedback-in #4(w428) -> ()
                    n132 = feedback #5(w425) -> (w441:u64)
                    n133 = Select(t=w425, s=w442, f=w441) -> (s? t:f=w437:u64)
                    n134 = Increment(x=w437) -> (x+1=w438:u64)
                    n135 = Select(t=w437, s=w429, f=w438) -> (s? t:f=w436:u64)
                    n136 = Greater?(x="Number of scans", y=w436) -> (0:w422:bool)
                    n137 = Multiply(x="Scan freq.  increment", y=w432) -> (x*y=w457:i64)
                    n138 = Select(t=TRUE, s="Cont. Scan", f=w422) -> (s? t:f=w421:bool)
                    "Scanning" <- w421
                    n139 = Select(t=w436, s=w421, f=w425) -> (s? t:f=w439:u64)
                    n140 = feedback-in #5(w439) -> ()
                    n141 = Increment(x=w436) -> (x+1=→"Scan I":u64)
                  }
                }
                n142 = feedback #6(w284) -> (w283:u16)
                n143 = Increment(x=w283) -> (x+1=w285:u16)
                n144 = Greater Or Equal?(x=w285, y="Trap Pos FB Int Count") -> (x >= y?=w276:bool)
                n145 = Select(t=w284, s=w276, f=w285) -> (s? t:f=w286:u16)
                n146 = feedback-in #6(w286) -> ()
                n147 = feedback #7(w291) -> (w290:fxp<+/-,24,9>)
                n148 = Add(x=w289, y=w290) -> (x+y=w282:fxp<+/-,24,9>)
                n149 = case "For intensity feedback" shown="True" "FB On/Off Set 1" {
                  tunnel: "BD 1 Amplitude 1" -> [w459 _]
                  tunnel: [w459 w463] -> w300
                  tunnel: w275 -> [_ w460]
                  tunnel: w274 -> [_ w461]
                  frame False {
                  }
                  frame True {
                    n150 = local read "AI2 Y Sum Set 1"() -> (w464:i16)
                    n151 = call "Slower PID.vi"("process variable"=w464, "reset?"="FB Reset Set 1", "setpoint"="FB Setpoint Set 1", "PID gains (x 2^8)"=w461, "output range"=w460) -> ("output"=w465:i16)  [unwired: 10 out]
                    n152 = To Unsigned Word Integer(number=w465) -> (unsigned 16bit integer=w463:u16)
                  }
                }
                n153 = Select(t=w291, s=w276, f=w282) -> (s? t:f=w294:fxp<+/-,24,9>)
                n154 = feedback-in #7(w294) -> ()
                n155 = Divide(x=w282, y="Trap Pos FB Int Count") -> (x/y=w277:fxp<+/-,16,1>)
                n156 = feedback #8(fxp<+/-,24,9> 0.0 ("AI1 X Set 2")) -> (w295:fxp<+/-,24,9>)
                n157 = Select(t=w282, s=w276, f=w295) -> (s? t:f=w296:fxp<+/-,24,9>)
                "Trap Pos FB Int Signal" <- w296
                n158 = feedback-in #8(w296) -> ()
                n159 = feedback #9(fxp<+/-,16,1> 0.0 ("Trap Pos FB Int-Norm Signal")) -> (w279:fxp<+/-,16,1>)
                n160 = Select(t=w277, s=w276, f=w279) -> (s? t:f=w278:fxp<+/-,16,1>)
                "Trap Pos FB Int-Norm Signal" <- w278
                n161 = feedback-in #9(w278) -> ()
                n162 = case "For position feedback" shown="True" "Force feedback" {
                  tunnel: [i64 0 w337] -> w297
                  tunnel: w277 -> [_ w334]
                  tunnel: w276 -> [_ w333]
                  frame False {
                  }
                  frame True {
                    n163 = feedback #10(i64 0) -> (w336:i64)
                    n164 = case shown="True" w333 {
                      tunnel: [w338 w352] -> w337
                      tunnel: w336 -> [w338 _]
                      tunnel: w334 -> [_ w346]
                      frame False {
                      }
                      frame True {
                        w356 = u32 0
                        n165 = Bundle("P2"="P2", "I2"="I2", "D2"="D2") -> (w342:T8)  [unwired: 1 in]
                        n166 = Bundle("FB2 output high"="FB2 output high", "FB2 output low"="FB2 output low") -> (w339:T9)  [unwired: 1 in]
                        n167 = xnode ("PID")("process variable"=w346, "reset?"="Trap Pos. FB Reset", "setpoint"="Trap Pos. FB SP", "PID gains"=w342, "output range"=w339) -> ("output"=w368:fxp<+/-,16,1>)
                        n168 = Negate(x=w368) -> (-x=w367:fxp<+/-,17,2>)
                        n169 = Select(t=w367, s="Trap Pos FB Negate Action", f=w368) -> (s? t:f=w364:fxp<+/-,17,2>)
                        n170 = Scale By Power Of 2(n=u32 15, x=u32 1) -> (x*2^n=w361:u32)
                        n171 = Multiply(x=w364, y=w361) -> (x*y=w360:fxp<+/-,17,17>)
                        n172 = To Quad Integer(1:w360) -> (0:w372:i64)
                        "Trap Pos FB Action" <- w372
                        n173 = Multiply(x=w372, y="Trap Pos. FB Mult Factor") -> (x*y=w370:i64)
                        n174 = Add(x=w370, y="Trap Pos. FB Offset Factor") -> (x+y=w352:i64)
                        n175 = feedback #11() -> (w353:i64)  [unwired: 1 in]
                        n176 = Add(x=w352, y=w353) -> (x+y=w350:i64)
                        n177 = feedback #12(w356) -> (w358:u32)
                        n178 = Increment(x=w358) -> (x+1=w347:u32)
                        n179 = Greater Or Equal?(x=w347, y="FB Trig Integrate") -> (x >= y?=w348:bool)
                        n180 = Select(t=i64 0, s=w348, f=w350) -> (s? t:f=w354:i64)
                        n181 = feedback-in #11(w354) -> ()
                        n182 = Select(t=w356, s=w348, f=w347) -> (s? t:f=w357:u32)
                        n183 = feedback-in #12(w357) -> ()
                        n184 = And(x=w348, y="FPGA Trap Trig") -> (x .and. y?=w355:bool)
                        n185 = case "Trap FB trigger excitation laser ON" shown="True" w355 {
                          tunnel: w350 -> [_ w376]
                          tunnel: w347 -> [_ w374]
                          frame False {
                          }
                          frame True {
                            n186 = Not(x="TTrig Negate Pos") -> (.not. x?=w383:bool)
                            n187 = Boolean To (0,1)(Boolean="TTrig Negate Pos") -> (0, 1=w381:i16)
                            n188 = Boolean To (0,1)(Boolean=w383) -> (0, 1=w382:i16)
                            n189 = Negate(x=w381) -> (-x=w380:i16)
                            n190 = Add(x=w380, y=w382) -> (x+y=w379:i16)
                            n191 = Multiply(x=w379, y=w376) -> (x*y=w378:i64)
                            "TTrig Sig" <- w378
                            n192 = Multiply(x="FPGA TTrig Thresh", y=w374) -> (x*y=w375:i64)
                            "TTrig Fin Thresh" <- w375
                            n193 = Greater Or Equal?(x=w378, y=w375) -> (x >= y?=w377:bool)
                            n194 = case shown="True" w377 {
                              frame False {
                              }
                              frame True {
                                w386 = TRUE ("Green FB On/Off")
                                w388 = u8 2 ("Operating Mode")
                                n195 = local write "Operating Mode 2"(w388) -> ()
                                n196 = local write "Operating Mode"(w388) -> ()
                                n197 = local write "Green FB On/Off"(w386) -> ()
                                n198 = local write "FPGA Trap Trig"(FALSE ("FPGA Trap Trig")) -> ()
                                "TTrig?" <- w386
                              }
                            }
                          }
                        }
                      }
                    }
                    n199 = feedback-in #10(w337) -> ()
                  }
                }
                n200 = Select(t=w307, s="Scan BD", f=w308) -> (s? t:f=w306:u64)
                n201 = Select(t=w308, s="Scan BD", f=w307) -> (s? t:f=w309:u64)
                n202 = Add(x=w306, y="BD 2 Frequency 1") -> (x+y=w311:u64)
                n203 = Compound Arithmetic op=ADD(i64 0 ("f"), "BD 1 Frequency 1", w297, w309) -> (w312:u64)
                "BD1 Frequency Out 1" <- w312
              }
              frame 2 {
                # "Trap 2"
                n204 = case shown="True" "FB On/Off Set 2" {
                  tunnel: [w477 w480] -> w473
                  tunnel: "BD 1 Amplitude 2" -> [w477 _]
                  tunnel: w470 -> [_ w479]
                  tunnel: w469 -> [_ w478]
                  frame False {
                  }
                  frame True {
                    n205 = local read "AI2 Y Sum Set 2"() -> (w483:i16)
                    n206 = call "Slower PID.vi"("process variable"=w483, "reset?"="FB Reset Set 2", "setpoint"="FB Setpoint Set 2", "PID gains (x 2^8)"=w479, "output range"=w478) -> ("output"=w481:i16)  [unwired: 10 out]
                    n207 = To Unsigned Word Integer(number=w481) -> (unsigned 16bit integer=w480:u16)
                  }
                }
                n208 = Add(x="BD 1 Frequency 2", y=i64 0 ("f")) -> (x+y=w468:u64)
                "BD1 Frequency Out 2" <- w468
              }
              frame 3 {
                # "Fluorescence period"
              }
            }
            n209 = feedback-in #13(w186) -> ()
            n210 = feedback #13(w186) -> (w185:u16)
            n211 = Select(t=w188, s="Interlace ON/OFF", f="Interlace Off Parameters") -> (s? t:f=w225:u8)
            n212 = Subtract(x=w186, y=w185) -> (x-y=w184:u16)
            n213 = Subtract "The error"(x=w184, y=w183) -> (x-y=w161:u16)
            n214 = case shown="1, Default" w225 {
              tunnel: ["DIO count 1 (ticks)" "DIO count 2 (ticks)" "DIO count 3 (ticks)"] -> w182
              frame 1, Default {
              }
              frame 2 {
              }
              frame 3 {
              }
            }
            n215 = Number To Boolean Array(number=w161) -> (Boolean array=w162:bool[])
            n216 = Or Array Elements(Boolean array=w162) -> (logical OR=w160:bool)
            n217 = Boolean To (0,1)(Boolean=w160) -> (0, 1=w167:i16)
            n218 = To Unsigned Byte Integer(number=w167) -> (unsigned 8bit integer=w164:u8)
            n219 = feedback #14(u8 0) -> (w165:u8)
            n220 = Add(x=w164, y=w165) -> (x+y=w163:u8)
            "DIO Late Counter" <- w163
            n221 = feedback-in #14(w163) -> ()
            n222 = Subtract(x=w182, y=w161) -> (x-y=w181:u16)
            n223 = Split Number(x=w222) -> (hi(x)=w221:u32, lo(x)=w220:u32)
            n224 = Split Number(x=w211) -> (hi(x)=w216:u32, lo(x)=w215:u32)
            n225 = Boolean To (0,1)(Boolean="+ phase (DIO)") -> (0, 1=w178:i16)
            n226 = Split Number(x=w221) -> (lo(x)=w219:u16)  [unwired: 1 out]
            n227 = Split Number(x=w220) -> (hi(x)=w218:u16, lo(x)=w217:u16)
            n228 = Split Number(x=w216) -> (lo(x)=w214:u16)  [unwired: 1 out]
            n229 = Split Number(x=w215) -> (hi(x)=w213:u16, lo(x)=w212:u16)
            n230 = Split Number(x=w171) -> (hi(x)=w173:u8, lo(x)=w172:u8)
            n231 = Split Number(x=w168) -> (hi(x)=w170:u8, lo(x)=w169:u8)
            n232 = Split Number(x=w219) -> (hi(x)=w210:u8, lo(x)=w209:u8)
            n233 = Split Number(x=w218) -> (hi(x)=w208:u8, lo(x)=w207:u8)
            n234 = Split Number(x=w214) -> (hi(x)=w203:u8, lo(x)=w202:u8)
            n235 = Split Number(x=w217) -> (hi(x)=w206:u8, lo(x)=w205:u8)
            n236 = Split Number(x=w213) -> (hi(x)=w201:u8, lo(x)=w200:u8)
            n237 = Split Number(x=w212) -> (hi(x)=w199:u8, lo(x)=w198:u8)
            n238 = Multiply(x=w178, y="Phase count adjustment (DIO)") -> (x*y=w174:i16)
            n239 = feedback #15(i16 0) -> (w176:i16)
            n240 = Subtract(x=w176, y=w174) -> (x-y=w175:i16)
            "DIO Relative phase" <- w175
            n241 = feedback-in #15(w175) -> ()
            n242 = Add(x=w181, y=w174) -> (x+y=w180:u16)
            n243 = Build Array "BD 1 A Stack"(w173, w172) -> (w195:u8[])
            n244 = Build Array "BD 2 A Stack"(w170, w169) -> (w194:u8[])
            n245 = Build Array "BD 1 nu Stack"(w210, w209, w208, w207, w206, w205) -> (w204:u8[])
            n246 = Build Array "BD 2 nu Stack"(w203, w202, w201, w200, w199, w198) -> (w197:u8[])
            n247 = case shown="2" w152 {
              tunnel: [w265 w268] -> w193
              tunnel: [u8 10 u8 4] -> w196
              tunnel: "Swap F1 and F2" -> [w266 w268]
              frame 2 {
                # "F2"
                n248 = Not(x=w266) -> (.not. x?=w265:bool)
              }
              frame 1, Default {
                # "low chooses F1"
                # "F1"
              }
            }
            n249 = case "If FPGA is controlling (toggling) RF synth" shown="True" w192 {
              tunnel: w204 -> [_ w241]
              tunnel: w197 -> [_ w240]
              tunnel: w196 -> [_ w239]
              tunnel: w195 -> [_ w238]
              tunnel: w194 -> [_ w237]
              frame False {
              }
              frame True {
                # "Write next amp.\n(wait until beginning of next loop iteration to update)"
                n250 = flat-sequence "Update the next F1 and F2 frequency value (the actual frequency won't change until FSK is switched).\nThen load the next amplitude value into buffer, but don't update it until the next cycle." {
                  tunnel: w240 -> [w243]
                  tunnel: w241 -> [w244]
                  tunnel: [w244] -> w236
                  tunnel: [w243] -> w235
                  tunnel: w239 -> [w245]
                  tunnel: w236 -> [w247]
                  tunnel: w235 -> [w246]
                  tunnel: w238 -> [w258]
                  tunnel: w237 -> [w257]
                  frame #0 {
                    # "To possibly send\nthese writes to very\nend of loop (for x and\ny phase adjust)"
                    n251 = call "Wait8"("Count(Ticks)"="Next trap write delay (ticks)") -> ()  [unwired: 1 out]
                  }
                  frame #1 {
                    n252 = for {
                      tunnel: w247 -> [w253] mode=indexing
                      tunnel: w246 -> [w252] mode=indexing
                      tunnel: w245 -> [w250]
                      i -> [w251]
                      # "Write next freq."
                      n253 = To Unsigned Byte Integer(number=w251) -> (unsigned 8bit integer=w248:u8)
                      n254 = Add(x=w250, y=w248) -> (x+y=w249:u8)
                      n255 = call "write to RF synth bd.vi"("Address Byte"=w249, "BD 2 Byte"=w252, "BD 1 Byte"=w253) -> ()
                    }
                  }
                  frame #2 {
                    w254 = TRUE ("Connector1/DIO15")
                    # "send udclk high\n(BD 1 and 2)"
                    n256 = xnode "FPGA I/O Node"("Connector1/DIO30"=w254, "Connector1/DIO29"=w254) -> ()  [unwired: 2 in, 2 out]
                  }
                  frame #3 {
                    w255 = FALSE ("Connector1/DIO15")
                    n257 = xnode "FPGA I/O Node"("Connector1/DIO30"=w255, "Connector1/DIO29"=w255) -> ()  [unwired: 2 in, 2 out]
                  }
                  frame #4 {
                    n258 = for {
                      tunnel: w258 -> [w264] mode=indexing
                      tunnel: w257 -> [w263] mode=indexing
                      tunnel: u8 33 -> [w261]
                      i -> [w262]
                      n259 = To Unsigned Byte Integer(number=w262) -> (unsigned 8bit integer=w259:u8)
                      n260 = Add(x=w261, y=w259) -> (x+y=w260:u8)
                      n261 = call "write to RF synth bd.vi"("Address Byte"=w260, "BD 2 Byte"=w263, "BD 1 Byte"=w264) -> ()
                    }
                  }
                }
              }
            }
          }
        }
      }
    }
  }
  n262 = while "APD 1 Counter" {
    tunnel: w2 -> [_]
    stop <- FALSE stop-if-true
    n263 = flat-sequence {
      frame #0 {
        n264 = xnode "FPGA I/O Method Node"("FPGA I/O In"=refnum<k21> "Connector0/DIO0" ("APD 1 DO"), "Timeout"=-1) -> ()  [unwired: 2 out]
      }
      frame #1 {
        n265 = local read "APD1 int gate"() -> (w492:bool)
        n266 = case shown="True" w492 {
          frame False {
          }
          frame True {
            n267 = local read "APD1 out state"() -> (w493:bool)
            n268 = case shown="True" w493 {
              frame False {
                n269 = local read "APD 1 Counts 0"() -> (w495:u32)
                n270 = Increment(x=w495) -> (x+1=→"APD 1 Counts 0":u32)
              }
              frame True {
                n271 = local read "APD 1 Counts 1"() -> (w497:u32)
                n272 = Increment(x=w497) -> (x+1=→"APD 1 Counts 1":u32)
              }
            }
          }
        }
      }
    }
  }
  n273 = while "Handshake memory transfer for trap oscillation sin wave data" {
    shift-right: [w499] -> _
    shift-left: w1 -> [w500]
    stop <- FALSE stop-if-true
    # "Write"
    n274 = case shown="1" w500 {
      tunnel: [w503 w508 w509] -> w499
      frame 3, Default {
        w501 = i16 2 items=["UnSet Ready", "ReadWrite", "Wait Ready"]
        w502 = i16 1 items=["UnSet Ready", "ReadWrite", "Wait Ready"]
        n275 = Select(t=w502, s="Ready Write", f=w501) -> (s? t:f=w503:i16)
      }
      frame 1 {
        w508 = i16 0 items=["UnSet Ready", "ReadWrite", "Wait Ready"]
        n276 = xnode ("Memory Write")("Address"="Address 2", "Data"="Data", "Memory In"=refnum<k21> "Trap osc memory") -> ()  [unwired: 1 out]
      }
      frame 0 {
        w509 = i16 2 items=["UnSet Ready", "ReadWrite", "Wait Ready"]
        n277 = local write "Ready Write"(FALSE ("Ready Read")) -> ()
      }
    }
  }
  n278 = while "APD 2 Counter" {
    tunnel: w2 -> [_]
    stop <- FALSE stop-if-true
    n279 = flat-sequence {
      frame #0 {
        n280 = xnode "FPGA I/O Method Node"("FPGA I/O In"=refnum<k21> "Connector0/DIO1" ("APD 2 DO"), "Timeout"=-1) -> ()  [unwired: 2 out]
      }
      frame #1 {
        n281 = local read "APD2 int gate"() -> (w514:bool)
        n282 = case shown="True" w514 {
          frame False {
          }
          frame True {
            n283 = local read "APD2 out state"() -> (w515:bool)
            n284 = case shown="False" w515 {
              frame False {
                n285 = local read "APD 2 Counts 0"() -> (w517:u32)
                n286 = Increment(x=w517) -> (x+1=→"APD 2 Counts 0":u32)
              }
              frame True {
                n287 = local read "APD 2 Counts 1"() -> (w519:u32)
                n288 = Increment(x=w519) -> (x+1=→"APD 2 Counts 1":u32)
              }
            }
          }
        }
      }
    }
  }
  n289 = while "APD 2 Gating" {
    shift-right: [w523] -> _
    shift-left: w2 -> [w528]
    shift-right: [w522] -> _
    shift-left: w6 -> [w520]
    stop <- FALSE stop-if-true
    n290 = flat-sequence {
      tunnel: w528 -> [w531]
      tunnel: [w532] -> w526
      tunnel: [w531] -> w524
      tunnel: [w530] -> w521
      tunnel: w520 -> [w530]
      tunnel: [w535] -> w527
      tunnel: w526 -> [w535]
      tunnel: [w534] -> w525
      tunnel: w524 -> [w534]
      tunnel: w521 -> [w533]
      tunnel: [w557] -> w523
      tunnel: w527 -> [w567]
      tunnel: w525 -> [w565]
      tunnel: [w536] -> w522
      frame #0 {
        n291 = call "Loop Timer8"("Count(Ticks)"=w531) -> ("Tick Count(Ticks)"=w532:u16)
      }
      frame #1 {
        # "Signal maybe then sent through \na transistor before APD"
        n292 = xnode "FPGA I/O Node"("Connector0/DIO8"=w533, "Connector0/DIO9"=w533, "Connector0/DIO10"=w533, "Connector0/DIO11"=w533) -> ()  [unwired: 4 in, 4 out]
        "APD2 int gate" <- w533
      }
      frame #2 {
        n293 = local read "APD Gate ON Count"() -> (w550:u16)
        n294 = local read "APD Gate OFF Count"() -> (w549:u16)
        n295 = feedback #16(TRUE) -> (w562:bool)
        n296 = feedback-in #17(w567) -> ()
        n297 = feedback #17(w567) -> (w551:u16)
        n298 = Not(x=w562) -> (.not. x?=w560:bool)
        n299 = feedback-in #16(w560) -> ()
        n300 = Subtract(x=w567, y=w551) -> (x-y=w566:u16)
        n301 = Select(t=w550, s=w560, f=w549) -> (s? t:f=w564:u16)
        n302 = Subtract(x=w566, y=w565) -> (x-y=w542:u16)
        n303 = Subtract(x=w564, y=w542) -> (x-y=w556:u16)
        n304 = Number To Boolean Array(number=w542) -> (Boolean array=w541:bool[])
        n305 = Or Array Elements(Boolean array=w541) -> (logical OR=w540:bool)
        n306 = Boolean To (0,1)(Boolean="+ phase (APD 2 Gate)") -> (0, 1=w554:i16)
        n307 = Multiply(x=w554, y="Phase count adjustment (APD 2 Gate)") -> (x*y=w552:i16)
        n308 = Boolean To (0,1)(Boolean=w540) -> (0, 1=w547:i16)
        n309 = Add(x=w556, y=w552) -> (x+y=w557:u16)
        n310 = To Unsigned Byte Integer(number=w547) -> (unsigned 8bit integer=w544:u8)
        n311 = feedback #18(i16 0) -> (w559:i16)
        n312 = Subtract(x=w559, y=w552) -> (x-y=w558:i16)
        "APD 2 Gate Relative Phase" <- w558
        n313 = feedback-in #18(w558) -> ()
        n314 = feedback #19(u8 0) -> (w545:u8)
        n315 = Add(x=w544, y=w545) -> (x+y=w543:u8)
        "APD 2 Gate Late Counter" <- w543
        n316 = feedback-in #19(w543) -> ()
        n317 = local read "APD Gate Operating Mode"() -> (w548:u8)
        n318 = case shown="2" w548 {
          tunnel: [TRUE FALSE w570] -> w537
          tunnel: w562 -> [_ _ w570]
          frame 0, Default {
          }
          frame 1 {
          }
          frame 2 {
          }
        }
        n319 = local read "Invert APD Gate"() -> (w539:bool)
        n320 = Not(x=w537) -> (.not. x?=w538:bool)
        n321 = Select(t=w538, s=w539, f=w537) -> (s? t:f=w536:bool)
      }
    }
  }
  n322 = while "532 nm green fluorescent laser interlacing (DO to IA 532 nm AOM ME amp)." {
    shift-right: [w574] -> _
    shift-left: w2 -> [w579]
    shift-right: [w573] -> _
    shift-left: w3 -> [w571]
    stop <- FALSE stop-if-true
    n323 = flat-sequence {
      tunnel: w579 -> [w582]
      tunnel: [w583] -> w577
      tunnel: [w582] -> w575
      tunnel: [w581] -> w572
      tunnel: w571 -> [w581]
      tunnel: [w586] -> w578
      tunnel: w577 -> [w586]
      tunnel: [w585] -> w576
      tunnel: w575 -> [w585]
      tunnel: w572 -> [w584]
      tunnel: [w595] -> w574
      tunnel: w578 -> [w615]
      tunnel: w576 -> [w612]
      tunnel: [w604] -> w573
      frame #0 {
        n324 = call "Loop Timer4"("Count(Ticks)"=w582) -> ("Tick Count(Ticks)"=w583:u16)
      }
      frame #1 {
        n325 = xnode "FPGA I/O Node"("Connector1/DIO34"=w584, "Connector1/DIO38"=w584, "Connector1/DIO39"=w584) -> ()  [unwired: 3 in, 3 out]
      }
      frame #2 {
        n326 = feedback-in #20(w615) -> ()
        n327 = feedback #20(w615) -> (w614:u16)
        n328 = Subtract(x=w615, y=w614) -> (x-y=w613:u16)
        n329 = Subtract(x=w613, y=w612) -> (x-y=w588:u16)
        n330 = Number To Boolean Array(number=w588) -> (Boolean array=w589:bool[])
        n331 = Or Array Elements(Boolean array=w589) -> (logical OR=w587:bool)
        n332 = Boolean To (0,1)(Boolean="+ phase (GI)") -> (0, 1=w600:i16)
        n333 = Multiply(x=w600, y="Phase count adjustment (GI)") -> (x*y=w597:i16)
        n334 = Boolean To (0,1)(Boolean=w587) -> (0, 1=w594:i16)
        n335 = To Unsigned Byte Integer(number=w594) -> (unsigned 8bit integer=w591:u8)
        n336 = feedback #21(i16 0) -> (w598:i16)
        n337 = feedback #22(u8 0) -> (w592:u8)
        n338 = Add(x=w591, y=w592) -> (x+y=w590:u8)
        "GI Late Counter" <- w590
        n339 = feedback-in #22(w590) -> ()
        n340 = Subtract(x=w598, y=w597) -> (x-y=w596:i16)
        "GI Relative phase" <- w596
        n341 = feedback-in #21(w596) -> ()
        n342 = feedback #23(TRUE) -> (w607:bool)
        n343 = case shown="2" "Operating Mode" {
          tunnel: [TRUE FALSE w621] -> w604
          tunnel: w607 -> [_ _ w618]
          frame 0, Default {
          }
          frame 1 {
          }
          frame 2 {
            n344 = Not(x=w618) -> (.not. x?=w620:bool)
            n345 = Select(t=w620, s="Invert GI", f=w618) -> (s? t:f=w621:bool)
          }
        }
        n346 = Not(x=w607) -> (.not. x?=w603:bool)
        n347 = Select(t="Green interlace ON count", s=w603, f="Green interlace OFF count") -> (s? t:f=w609:u16)
        n348 = Subtract(x=w609, y=w588) -> (x-y=w601:u16)
        n349 = Add(x=w601, y=w597) -> (x+y=w595:u16)
        n350 = feedback-in #23(w603) -> ()
      }
    }
  }
  n351 = while "Green and red fluorescent laser interlacing (Current AO to IA 532 nm AOM ME amp)." {
    shift-right: [w630] -> _
    shift-left: w2 -> [w633]
    shift-right: [w627] -> _
    shift-left: w4 -> [w625]
    shift-right: [w624] -> _
    shift-left: w4 -> [w623]
    stop <- FALSE stop-if-true
    n352 = flat-sequence {
      tunnel: w633 -> [w637]
      tunnel: [w638] -> w632
      tunnel: [w637] -> w631
      tunnel: [w636] -> w626
      tunnel: w625 -> [w636]
      tunnel: w623 -> [w635]
      tunnel: [w635] -> w622
      tunnel: [w642] -> w629
      tunnel: w632 -> [w642]
      tunnel: [w641] -> w628
      tunnel: w631 -> [w641]
      tunnel: w626 -> [w640]
      tunnel: w622 -> [w639]
      tunnel: [w663] -> w630
      tunnel: [w679] -> w627
      tunnel: w629 -> [w690]
      tunnel: w628 -> [w687]
      tunnel: [w647] -> w624
      frame #0 {
        n353 = call "Loop Timer10"("Count(Ticks)"=w637) -> ("Tick Count(Ticks)"=w638:u16)
      }
      frame #1 {
        n354 = xnode "FPGA I/O Node"("Chassis2/Mod1/AO0"=w640, "Chassis2/Mod1/AO1"=w639) -> ()  [unwired: 2 in, 2 out]
      }
      frame #2 {
        # "Design note:\n\nThese two laser controls are in the same loop\nbecause the expansion current AI cannot separately\ntime the outputs fast enough for us.  Apparently\nit is because of communication time between the\nexpansion card and the fpga.\n\nSo the two analog control signals have the same timing\nand profile, but independent amplitudes to independently\ncontrol the intensity and feedback for each laser."
        n355 = feedback #24(TRUE) -> (w643:bool)
        n356 = Not(x=w643) -> (.not. x?=w644:bool)
        n357 = feedback-in #24(w644) -> ()
        n358 = Subtract(x="Green interlace OFF count 2", y="Green int current ON count adj") -> (x-y=w672:u16)
        n359 = feedback-in #25(w690) -> ()
        n360 = feedback #25(w690) -> (w689:u16)
        n361 = Add(x="Green int current ON count adj", y="Green interlace ON count 2") -> (x+y=w673:u16)
        n362 = Subtract(x=w690, y=w689) -> (x-y=w688:u16)
        n363 = Select(t=w673, s=w644, f=w672) -> (s? t:f=w684:u16)
        n364 = Subtract(x=w688, y=w687) -> (x-y=w656:u16)
        n365 = case shown="2" "RI Operating Mode 2" {
          tunnel: [TRUE FALSE w696] -> w645
          tunnel: w643 -> [_ _ w693]
          frame 0, Default {
          }
          frame 1 {
          }
          frame 2 {
            n366 = Not(x=w693) -> (.not. x?=w695:bool)
            n367 = Select(t=w695, s="Invert RI 2", f=w693) -> (s? t:f=w696:bool)
          }
        }
        n368 = Subtract(x=w684, y=w656) -> (x-y=w667:u16)
        n369 = case shown="0, Default" "Operating Mode 2" {
          tunnel: [TRUE FALSE w730] -> w648
          tunnel: w643 -> [_ _ w727]
          frame 0, Default {
          }
          frame 1 {
          }
          frame 2 {
            n370 = Not(x=w727) -> (.not. x?=w729:bool)
            n371 = Select(t=w729, s="Invert GI 2", f=w727) -> (s? t:f=w730:bool)
          }
        }
        n372 = Number To Boolean Array(number=w656) -> (Boolean array=w657:bool[])
        n373 = Boolean To (0,1)(Boolean="+ phase (GI) 2") -> (0, 1=w669:i16)
        n374 = Or Array Elements(Boolean array=w657) -> (logical OR=w655:bool)
        n375 = Boolean To (0,1)(Boolean=w655) -> (0, 1=w662:i16)
        n376 = Multiply(x=w669, y="Phase count adjustment (GI) 2") -> (x*y=w665:i16)
        n377 = To Unsigned Byte Integer(number=w662) -> (unsigned 8bit integer=w658:u8)
        n378 = Add(x=w667, y=w665) -> (x+y=w663:u16)
        n379 = feedback #26(u8 0) -> (w660:u8)
        n380 = Add(x=w658, y=w660) -> (x+y=w659:u8)
        "GI Late Counter 2" <- w659
        n381 = feedback-in #26(w659) -> ()
        n382 = feedback #27(i16 0) -> (w666:i16)
        n383 = Subtract(x=w666, y=w665) -> (x-y=w664:i16)
        "GI Relative phase 2" <- w664
        n384 = feedback-in #27(w664) -> ()
        n385 = And(x=w648, y="Green FB On/Off") -> (x .and. y?=w674:bool)
        n386 = And(x=w645, y="Red FB On/Off") -> (x .and. y?=w654:bool)
        n387 = case shown="False" w674 {
          tunnel: "Current Out" -> [w711 _]
          tunnel: [w711 w720] -> w678
          frame False {
          }
          frame True {
            n388 = local read "Green FB Sum"() -> (w716:i16)
            n389 = Bundle("P3"="P3", "I3"="I3", "D3"="D3") -> (w712:cluster{"P3":i16, "I3":i16, "D3":i16})  [unwired: 1 in]
            n390 = call "Slower PID.vi"("process variable"=w716, "reset?"="Green FB Reset", "setpoint"="Green FB Setpoint", "PID gains (x 2^8)"=w712, "output range"=cluster{"output high":i16, "output low":i16} {"output high"=32767, "output low"=-32768} ("Green FB output range")) -> ("output"=w723:i16)  [unwired: 10 out]
            n391 = To Long Integer(number=w723) -> (32bit integer=w717:i32)
            n392 = Add(x=w717, y=32768) -> (x+y=w719:i32)
            n393 = To Unsigned Word Integer(number=w719) -> (unsigned 16bit integer=w720:u16)
          }
        }
        n394 = case shown="True" w654 {
          tunnel: "RI Current Out" -> [w697 _]
          tunnel: [w697 w706] -> w650
          frame False {
          }
          frame True {
            n395 = local read "Red FB Intensity"() -> (w702:i16)
            n396 = Bundle("P4"="P4", "I4"="I4", "D4"="D4") -> (w698:cluster{"P4":i16, "I4":i16, "D4":i16})  [unwired: 1 in]
            n397 = call "Slower PID.vi"("process variable"=w702, "reset?"="Red FB Reset", "setpoint"="Red FB Setpoint", "PID gains (x 2^8)"=w698, "output range"=cluster{"output high":i16, "output low":i16} {"output high"=32767, "output low"=-32768} ("Green FB output range")) -> ("output"=w709:i16)  [unwired: 10 out]
            n398 = To Long Integer(number=w709) -> (32bit integer=w703:i32)
            n399 = Add(x=w703, y=32768) -> (x+y=w705:i32)
            n400 = To Unsigned Word Integer(number=w705) -> (unsigned 16bit integer=w706:u16)
          }
        }
        n401 = Boolean To (0,1)(Boolean=w648) -> (0, 1=w680:i16)
        n402 = Boolean To (0,1)(Boolean=w645) -> (0, 1=w649:i16)
        n403 = To Unsigned Word Integer(number=w680) -> (unsigned 16bit integer=w677:u16)
        n404 = To Unsigned Word Integer(number=w649) -> (unsigned 16bit integer=w651:u16)
        n405 = Multiply(x=w677, y=w678) -> (x*y=w679:u16)
        n406 = Multiply(x=w651, y=w650) -> (x*y=w647:u16)
      }
    }
  }
  n407 = while "Excitation laser intensity feedback measurement (all lasers)" {
    shift-right: [w731] -> _
    shift-left: w2 -> [w736]
    stop <- FALSE stop-if-true
    n408 = flat-sequence {
      tunnel: w736 -> [w738]
      tunnel: [w739] -> w734
      tunnel: [w738] -> w732
      tunnel: [w745] -> w735
      tunnel: w734 -> [w745]
      tunnel: [w744] -> w733
      tunnel: w732 -> [w744]
      tunnel: [w757] -> w731
      tunnel: w735 -> [w768]
      tunnel: w733 -> [w765]
      frame #0 {
        n409 = call "Loop Timer9"("Count(Ticks)"=w738) -> ("Tick Count(Ticks)"=w739:u16)
      }
      frame #1 {
        # "Design note:\n\nAll lasers need to be measured at the same \ntime because the AI expansion module\ncannot independently time the measurements\nwithin our requirements: their is dead time.\n\nThis probably wouldn't be an issue with the built\nin AI on the fpga board itself."
        n410 = xnode "FPGA I/O Node"("Connector1/DIO35"=TRUE) -> ("Chassis2/Mod2/AI2"=→"Blue Intensity":i16, "Chassis2/Mod2/AI1"=→"Red FB Intensity":i16, "Chassis2/Mod2/AI0"=→"Green FB Sum":i16)  [unwired: 4 in, 4 out]
      }
      frame #2 {
        n411 = feedback-in #28(w768) -> ()
        n412 = feedback #28(w768) -> (w767:u16)
        n413 = Subtract(x=w768, y=w767) -> (x-y=w766:u16)
        n414 = xnode "FPGA I/O Node"("Connector1/DIO35"=FALSE) -> ()  [unwired: 1 in, 1 out]
        n415 = Subtract(x=w766, y=w765) -> (x-y=w747:u16)
        n416 = Subtract(x="Green FB Count", y=w747) -> (x-y=w761:u16)
        n417 = Number To Boolean Array(number=w747) -> (Boolean array=w748:bool[])
        n418 = Or Array Elements(Boolean array=w748) -> (logical OR=w746:bool)
        n419 = Boolean To (0,1)(Boolean="+ phase (Green FB)") -> (0, 1=w759:i16)
        n420 = Boolean To (0,1)(Boolean=w746) -> (0, 1=w753:i16)
        n421 = Multiply(x=w759, y="Phase count adjustment (Green FB)") -> (x*y=w754:i16)
        n422 = Add(x=w761, y=w754) -> (x+y=w757:u16)
        n423 = To Unsigned Byte Integer(number=w753) -> (unsigned 8bit integer=w750:u8)
        n424 = feedback #29(i16 0) -> (w756:i16)
        n425 = Subtract(x=w756, y=w754) -> (x-y=w755:i16)
        "Green FB Relative Phase" <- w755
        n426 = feedback-in #29(w755) -> ()
        n427 = feedback #30(u8 0) -> (w751:u8)
        n428 = Add(x=w750, y=w751) -> (x+y=w749:u8)
        "Green Late Counter" <- w749
        n429 = feedback-in #30(w749) -> ()
      }
    }
  }
  n430 = while "APD 1 Gating" {
    shift-right: [w772] -> _
    shift-left: w2 -> [w777]
    shift-right: [w771] -> _
    shift-left: w6 -> [w769]
    stop <- FALSE stop-if-true
    n431 = flat-sequence {
      tunnel: w777 -> [w780]
      tunnel: [w781] -> w775
      tunnel: [w780] -> w773
      tunnel: [w779] -> w770
      tunnel: w769 -> [w779]
      tunnel: [w784] -> w776
      tunnel: w775 -> [w784]
      tunnel: [w783] -> w774
      tunnel: w773 -> [w783]
      tunnel: w770 -> [w782]
      tunnel: [w802] -> w772
      tunnel: w776 -> [w816]
      tunnel: w774 -> [w813]
      tunnel: [w785] -> w771
      frame #0 {
        n432 = call "Loop Timer7"("Count(Ticks)"=w780) -> ("Tick Count(Ticks)"=w781:u16)
      }
      frame #1 {
        # "Signal maybe then sent through \na transistor before APD"
        n433 = xnode "FPGA I/O Node"("Connector0/DIO4"=w782, "Connector0/DIO5"=w782, "Connector0/DIO6"=w782, "Connector0/DIO7"=w782) -> ()  [unwired: 4 in, 4 out]
        "APD1 int gate" <- w782
      }
      frame #2 {
        n434 = feedback #31(TRUE) -> (w808:bool)
        n435 = feedback-in #32(w816) -> ()
        n436 = feedback #32(w816) -> (w815:u16)
        n437 = Not(x=w808) -> (.not. x?=w805:bool)
        n438 = feedback-in #31(w805) -> ()
        n439 = Subtract(x=w816, y=w815) -> (x-y=w814:u16)
        n440 = Select(t="APD Gate ON Count", s=w805, f="APD Gate OFF Count") -> (s? t:f=w810:u16)
        n441 = Subtract(x=w814, y=w813) -> (x-y=w790:u16)
        n442 = Subtract(x=w810, y=w790) -> (x-y=w801:u16)
        n443 = Number To Boolean Array(number=w790) -> (Boolean array=w791:bool[])
        n444 = Or Array Elements(Boolean array=w791) -> (logical OR=w789:bool)
        n445 = Boolean To (0,1)(Boolean="+ phase (APD 1 Gate)") -> (0, 1=w799:i16)
        n446 = Boolean To (0,1)(Boolean=w789) -> (0, 1=w796:i16)
        n447 = Multiply(x=w799, y="Phase count adjustment (APD 1 Gate)") -> (x*y=w797:i16)
        n448 = To Unsigned Byte Integer(number=w796) -> (unsigned 8bit integer=w793:u8)
        n449 = Add(x=w801, y=w797) -> (x+y=w802:u16)
        n450 = feedback #33(i16 0) -> (w804:i16)
        n451 = Subtract(x=w804, y=w797) -> (x-y=w803:i16)
        "APD 1 Gate Relative Phase" <- w803
        n452 = feedback-in #33(w803) -> ()
        n453 = feedback #34(u8 0) -> (w794:u8)
        n454 = Add(x=w793, y=w794) -> (x+y=w792:u8)
        "APD 1 Gate Late Counter" <- w792
        n455 = feedback-in #34(w792) -> ()
        n456 = case shown="2" "APD Gate Operating Mode" {
          tunnel: [TRUE FALSE w819] -> w786
          tunnel: w808 -> [_ _ w819]
          frame 0, Default {
          }
          frame 1 {
          }
          frame 2 {
          }
        }
        n457 = Not(x=w786) -> (.not. x?=w787:bool)
        n458 = Select(t=w787, s="Invert APD Gate", f=w786) -> (s? t:f=w785:bool)
      }
    }
  }
  n459 = while "MCL stage control" {
    shift-right: [w832] -> _
    shift-left: w2 -> [w835]
    shift-right: [w825] -> _
    shift-left: w11 -> [w822]
    shift-right: [w824] -> _
    shift-left: w10 -> [w820]
    stop <- FALSE stop-if-true
    n460 = flat-sequence {
      tunnel: w835 -> [w839]
      tunnel: [w840] -> w831
      tunnel: [w839] -> w829
      tunnel: [w838] -> w823
      tunnel: w822 -> [w838]
      tunnel: [w837] -> w821
      tunnel: w820 -> [w837]
      tunnel: w831 -> [w844]
      tunnel: [w844] -> w830
      tunnel: w829 -> [w843]
      tunnel: [w843] -> w828
      tunnel: w823 -> [w842]
      tunnel: w821 -> [w841]
      tunnel: w830 -> [w852]
      tunnel: w828 -> [w851]
      tunnel: [w852] -> w834
      tunnel: [w851] -> w833
      tunnel: [w850] -> w827
      tunnel: [w849] -> w826
      tunnel: [w924] -> w832
      tunnel: w834 -> [w931]
      tunnel: w833 -> [w928]
      tunnel: w827 -> [w926]
      tunnel: w826 -> [w925]
      tunnel: [w926] -> w825
      tunnel: [w925] -> w824
      frame #0 {
        n461 = call "Loop Timer5"("Count(Ticks)"=w839) -> ("Tick Count(Ticks)"=w840:u32)
      }
      frame #1 {
        n462 = xnode "FPGA I/O Node"("Connector0/AO1"=w842, "Connector0/AO2"=w841) -> ()  [unwired: 2 in, 2 out]
      }
      frame #2 {
        n463 = local read "Scanning MCL"() -> (w864:bool)
        n464 = Or(x=w864, y="Start scan (MCL)") -> (x .or. y?=w859:bool)
        n465 = Not(x="Abort scan (MCL)") -> (.not. x?=w857:bool)
        n466 = And(x=w857, y=w859) -> (x .and. y?=w856:bool)
        n467 = case "Raster scan" shown="True" w856 {
          tunnel: [w865 w908] -> w861
          tunnel: "Start scan (MCL)" -> [_ w893]
          tunnel: [w865 w869] -> w845
          frame False {
            w865 = i16 0
            n468 = local write "Scanning MCL"(FALSE ("scanning")) -> ()
          }
          frame True {
            w879 = i16 0
            w878 = u64 0
            # "scan incr."
            # "freq. incr. mult."
            # "count steps"
            # "count number of cycles"
            n469 = feedback #35(w878) -> (w905:u64)
            n470 = Select(t=w878, s=w893, f=w905) -> (s? t:f=w907:u64)
            n471 = Increment(x=w907) -> (x+1=w904:u64)
            n472 = Greater?(x="Cycles per step (MCL)", y=w904) -> (0:w888:bool)
            n473 = Select(t=w904, s=w888, f=w878) -> (s? t:f=w903:u64)
            n474 = feedback-in #35(w903) -> ()
            n475 = feedback #36(w878) -> (w902:u64)
            n476 = Select(t=w878, s=w893, f=w902) -> (s? t:f=w897:u64)
            n477 = Increment(x=w897) -> (x+1=w901:u64)
            n478 = Add(x="Scan steps (MCL)", y="Scan steps (MCL)") -> (x+y=w900:u64)
            n479 = Select(t=w897, s=w888, f=w901) -> (s? t:f=w883:u64)
            n480 = Greater?(x=w900, y=w883) -> (0:w882:bool)
            n481 = Select(t=w883, s=w882, f=w878) -> (s? t:f=w898:u64)
            n482 = feedback-in #36(w898) -> ()
            n483 = Equal?(x="Scan steps (MCL)", y=w883) -> (x = y?=w887:bool)
            n484 = Greater?(x="Scan steps (MCL)", y=w897) -> (0:w896:bool)
            n485 = feedback #37(w879) -> (w899:i16)
            n486 = Select(t=w879, s=w893, f=w899) -> (s? t:f=w885:i16)
            n487 = Increment(x=w885) -> (x+1=w895:i16)
            n488 = Decrement(x=w885) -> (x-1=w894:i16)
            n489 = Select(t=w895, s=w896, f=w894) -> (s? t:f=w886:i16)
            n490 = Select(t=w885, s=w887, f=w886) -> (s? t:f=w884:i16)
            n491 = Select(t=w885, s=w888, f=w884) -> (s? t:f=w880:i16)
            n492 = Select(t=w880, s=w882, f=w879) -> (s? t:f=w881:i16)
            n493 = feedback-in #37(w881) -> ()
            n494 = feedback #38(w878) -> (w892:u64)
            n495 = Select(t=w878, s=w893, f=w892) -> (s? t:f=w867:u64)
            n496 = Increment(x=w867) -> (x+1=w889:u64)
            n497 = Select(t=w867, s=w882, f=w889) -> (s? t:f=w868:u64)
            n498 = Greater?(x="Number of scans (MCL)", y=w868) -> (0:w875:bool)
            n499 = Multiply(x="Scan freq.  increment (MCL)", y=w885) -> (x*y=w908:i16)
            n500 = Select(t=TRUE, s="Cont. Scan (MCL)", f=w875) -> (s? t:f=w874:bool)
            "Scanning MCL" <- w874
            n501 = Select(t=w868, s=w874, f=w878) -> (s? t:f=w890:u64)
            n502 = feedback-in #38(w890) -> ()
            n503 = Increment(x=w868) -> (x+1=→"Scan I (MCL)":u64)
            n504 = To Word Integer(number=w867) -> (16bit integer=w870:i16)
            n505 = Multiply(x=w870, y="Scan freq.  increment (MCL)") -> (x*y=w869:i16)
          }
        }
        n506 = Select(t=w845, s="1D or 2D Scan?", f=i16 0) -> (s? t:f=w846:i16)
        n507 = Select(t=w846, s="MCL Scan Axis", f=w861) -> (s? t:f=w860:i16)
        n508 = Select(t=w861, s="MCL Scan Axis", f=w846) -> (s? t:f=w862:i16)
        n509 = Add(x=w860, y="AO2") -> (x+y=w849:i16)
        n510 = Add(x="AO1", y=w862) -> (x+y=w850:i16)
      }
      frame #3 {
        n511 = feedback-in #39(w931) -> ()
        n512 = feedback #39(w931) -> (w930:u32)
        n513 = Boolean To (0,1)(Boolean="+ phase (MCL)") -> (0, 1=w922:i16)
        n514 = Subtract(x=w931, y=w930) -> (x-y=w929:u32)
        n515 = Multiply(x=w922, y="Phase count adjustment (MCL)") -> (x*y=w918:i16)
        n516 = Subtract(x=w929, y=w928) -> (x-y=w910:u32)
        n517 = Subtract(x="MCL count", y=w910) -> (x-y=w920:u32)
        n518 = feedback #40(i16 0) -> (w919:i16)
        n519 = Subtract(x=w919, y=w918) -> (x-y=w917:i16)
        "MCL Relative Phase" <- w917
        n520 = feedback-in #40(w917) -> ()
        n521 = Number To Boolean Array(number=w910) -> (Boolean array=w911:bool[])
        n522 = Or Array Elements(Boolean array=w911) -> (logical OR=w909:bool)
        n523 = Boolean To (0,1)(Boolean=w909) -> (0, 1=w916:i16)
        n524 = Add(x=w920, y=w918) -> (x+y=w924:u32)
        n525 = To Unsigned Byte Integer(number=w916) -> (unsigned 8bit integer=w913:u8)
        n526 = feedback #41(u8 0) -> (w914:u8)
        n527 = Add(x=w913, y=w914) -> (x+y=w912:u8)
        "MCL Late Counter" <- w912
        n528 = feedback-in #41(w912) -> ()
      }
    }
  }
  n529 = while "Control APD data integration - stream to host" {
    shift-right: [w936] -> _
    shift-left: w7 -> [w941]
    stop <- FALSE stop-if-true
    n530 = flat-sequence {
      tunnel: w941 -> [w943]
      tunnel: [w944] -> w939
      tunnel: [w943] -> w937
      tunnel: [w954] -> w940
      tunnel: w939 -> [w954]
      tunnel: [w953] -> w938
      tunnel: w937 -> [w953]
      tunnel: [w952] -> w935
      tunnel: [w951] -> w934
      tunnel: [w945] -> w933
      tunnel: [w996] -> w936
      tunnel: w940 -> [w1006]
      tunnel: w938 -> [w1003]
      tunnel: w935 -> [w989]
      tunnel: w934 -> [w988]
      tunnel: w933 -> [w976]
      frame #0 {
        n531 = call "Loop Timer6"("Count(Ticks)"=w943) -> ("Tick Count(Ticks)"=w944:u32)
      }
      frame #1 {
        n532 = flat-sequence {
          tunnel: [w956] -> w950
          tunnel: w950 -> [w959]
          tunnel: [w963] -> w949
          tunnel: [w962] -> w948
          tunnel: [w959] -> w947
          tunnel: [w958] -> w946
          tunnel: [w970] -> w951
          tunnel: [w971] -> w952
          tunnel: w949 -> [w971]
          tunnel: w948 -> [w970]
          tunnel: w947 -> [w969]
          tunnel: w946 -> [w968]
          tunnel: [w968] -> w945
          frame #0 {
            # "use separate variable so each APD won't\nhave to wait to read"
            n533 = feedback #42(FALSE) -> (w955:bool)
            "APD1 out state" <- w955
            "APD2 out state" <- w955
            "APD3 out state" <- w955
            n534 = Not(x=w955) -> (.not. x?=w956:bool)
            n535 = feedback-in #42(w956) -> ()
          }
          frame #1 {
            n536 = local read "APD 3 Counts 1"() -> (w961:u32)
            n537 = local read "APD 3 Counts 0"() -> (w960:u32)
            n538 = local read "APD 1 Counts 1"() -> (w967:u32)
            n539 = local read "APD 1 Counts 0"() -> (w966:u32)
            n540 = local read "APD 2 Counts 1"() -> (w965:u32)
            n541 = local read "APD 2 Counts 0"() -> (w964:u32)
            n542 = Select(t=w961, s=w959, f=w960) -> (s? t:f=w958:u32)
            n543 = Select(t=w967, s=w959, f=w966) -> (s? t:f=w963:u32)
            n544 = Select(t=w965, s=w959, f=w964) -> (s? t:f=w962:u32)
          }
          frame #2 {
            n545 = case shown="False" w969 {
              frame False {
                w972 = u32 0 ("APD 1 Counts 0")
                n546 = local write "APD 1 Counts 0"(w972) -> ()
                n547 = local write "APD 2 Counts 0"(w972) -> ()
                n548 = local write "APD 3 Counts 0"(w972) -> ()
              }
              frame True {
                w973 = u32 0 ("APD 1 Counts 1")
                n549 = local write "APD 1 Counts 1"(w973) -> ()
                n550 = local write "APD 2 Counts 1"(w973) -> ()
                n551 = local write "APD 3 Counts 1"(w973) -> ()
              }
            }
          }
        }
      }
      frame #2 {
        n552 = feedback-in #43(w1006) -> ()
        n553 = feedback #43(w1006) -> (w1005:u32)
        n554 = Subtract(x=w1006, y=w1005) -> (x-y=w1004:u32)
        n555 = Subtract(x=w1004, y=w1003) -> (x-y=w981:u32)
        n556 = case shown="True" "APD to FIFO" {
          tunnel: w989 -> [_ w1011]
          tunnel: w988 -> [_ w1009]
          tunnel: w976 -> [_ w1007]
          frame False {
          }
          frame True {
            n557 = flat-sequence {
              tunnel: 0 ("Timeout") -> [w1013]
              tunnel: w1011 -> [w1014]
              tunnel: [w1013] -> w1010
              tunnel: w1010 -> [w1015]
              tunnel: w1009 -> [w1016]
              tunnel: [w1015] -> w1008
              tunnel: w1008 -> [w1018]
              tunnel: w1007 -> [w1017]
              frame #0 {
                n558 = xnode ("FIFO Write")("Element"=w1014, "Timeout"=w1013) -> ()  [unwired: 1 in, 2 out]
              }
              frame #1 {
                n559 = xnode ("FIFO Write")("Element"=w1016, "Timeout"=w1015) -> ()  [unwired: 1 in, 2 out]
              }
              frame #2 {
                n560 = xnode ("FIFO Write")("Element"=w1017, "Timeout"=w1018) -> ()  [unwired: 1 in, 2 out]
              }
            }
          }
        }
        n561 = Subtract(x="APD Acq Rate Count", y=w981) -> (x-y=w997:u32)
        n562 = Number To Boolean Array(number=w981) -> (Boolean array=w982:bool[])
        n563 = Or Array Elements(Boolean array=w982) -> (logical OR=w980:bool)
        n564 = Boolean To (0,1)(Boolean=w980) -> (0, 1=w987:i16)
        n565 = To Unsigned Byte Integer(number=w987) -> (unsigned 8bit integer=w984:u8)
        n566 = feedback #44(u8 0) -> (w985:u8)
        n567 = Add(x=w984, y=w985) -> (x+y=w983:u8)
        "APD Acq Late Counter" <- w983
        n568 = feedback-in #44(w983) -> ()
        n569 = Boolean To (0,1)(Boolean="+ phase (APD Acq)") -> (0, 1=w993:i16)
        n570 = Multiply(x=w993, y="Phase Count Adjustment (APD Acq)") -> (x*y=w990:i16)
        n571 = Add(x=w997, y=w990) -> (x+y=w996:u32)
        n572 = feedback #45(i16 0) -> (w995:i16)
        n573 = Subtract(x=w995, y=w990) -> (x-y=w992:i16)
        "APD Acq Relative Phase" <- w992
        n574 = feedback-in #45(w992) -> ()
        n575 = To Word Integer(number=w989) -> (16bit integer=w998:i16)
        n576 = To Word Integer(number=w976) -> (16bit integer=w977:i16)
        n577 = To Word Integer(number=w988) -> (16bit integer=w999:i16)
        n578 = Multiply(x="APD AO scale factor", y=w999) -> (x*y=w978:i16)
        n579 = Multiply(x="APD AO scale factor", y=w977) -> (x*y=w974:i16)
        n580 = Multiply(x="APD AO scale factor", y=w998) -> (x*y=w979:i16)
        n581 = xnode "FPGA I/O Node"("Connector0/AO6"=w979, "Connector0/AO7"=w978, "Connector0/AO5"=w974) -> ()  [unwired: 3 in, 3 out]
      }
    }
  }
  n582 = while "DAQ AI set 1" {
    shift-right: [w1019] -> _
    shift-left: w2 -> [w1024]
    stop <- FALSE stop-if-true
    n583 = flat-sequence {
      tunnel: w1024 -> [w1034]
      tunnel: [w1035] -> w1022
      tunnel: [w1034] -> w1021
      tunnel: [w1045] -> w1032
      tunnel: [w1044] -> w1031
      tunnel: [w1043] -> w1030
      tunnel: [w1042] -> w1029
      tunnel: [w1041] -> w1028
      tunnel: [w1040] -> w1027
      tunnel: [w1039] -> w1026
      tunnel: [w1038] -> w1025
      tunnel: [w1037] -> w1023
      tunnel: w1022 -> [w1037]
      tunnel: w1021 -> [w1036]
      tunnel: [w1036] -> w1020
      tunnel: [w1075] -> w1019
      tunnel: w1032 -> [w1101]
      tunnel: w1031 -> [w1067]
      tunnel: w1030 -> [w1068]
      tunnel: w1029 -> [w1047]
      tunnel: w1028 -> [w1091]
      tunnel: w1027 -> [w1090]
      tunnel: w1026 -> [w1089]
      tunnel: w1025 -> [w1088]
      tunnel: w1023 -> [w1085]
      tunnel: w1020 -> [w1082]
      frame #0 {
        n584 = call "Loop Timer3"("Count(Ticks)"=w1034) -> ("Tick Count(Ticks)"=w1035:u16)
      }
      frame #1 {
        n585 = xnode "FPGA I/O Node"("Connector1/DIO31"=TRUE ("Connector1/DIO33")) -> ("Connector0/AI0"=w1045:i16, "Connector0/AI1"=w1044:i16, "Connector0/AI2"=w1043:i16, "Connector0/AI3"=w1042:i16, "Connector0/AI4"=w1041:i16, "Connector0/AI5"=w1040:i16, "Connector0/AI6"=w1039:i16, "Connector0/AI7"=w1038:i16)  [unwired: 9 in, 9 out]
      }
      frame #2 {
        w1071 = FALSE ("AI to FIFO")
        # "Adjust phase after data acquired if button pressed"
        n586 = feedback #46(i16 1) -> (w1094:i16)
        n587 = Increment(x=w1094) -> (x+1=w1100:i16)
        n588 = Scale By Power Of 2(n="AI1 X Scale", x=w1067) -> (x*2^n=w1065:i16)
        n589 = Greater?(x=w1100, y="N of AI1 Int Acq Sets") -> (0:w1097:bool)
        n590 = Select(t=i16 1, s=w1097, f=w1100) -> (s? t:f=w1099:i16)
        n591 = feedback-in #46(w1099) -> ()
        n592 = Divide(x=w1065, y=w1047) -> (x/y=w1064:fxp<+/-,16,1>)
        n593 = feedback #47(w1071) -> (w1069:bool)
        n594 = feedback #48(w1071) -> (w1087:bool)
        n595 = case shown="2" w1094 {
          tunnel: w1068 -> [w1124 w1131 _]
          tunnel: ["Set 1" "Set 2" "Set 3"] -> w1092
          tunnel: ["AI to FIFO" w1133 w1138] -> w1086
          tunnel: w1087 -> [_ w1133 w1138]
          tunnel: ["Trap Pos to FIFO" w1132 w1137] -> w1070
          tunnel: w1069 -> [_ w1132 w1137]
          tunnel: w1064 -> [w1123 w1130 _]
          tunnel: [w1122 w1128 FALSE] -> w1051
          tunnel: [w1121 w1129 u64 0 ("BD1 Frequency Out 2")] -> w1050
          frame 1, Default {
            n596 = local read "BD1 Frequency Out 1"() -> (w1121:u64)
            n597 = Compound Arithmetic op=AND("Trap Pos to FIFO", "Set 1", "AI to FIFO") -> (w1122:bool)
            "AI2 Y Sum Set 1" <- w1124
            "AI1 X Set 1" <- w1123
          }
          frame 2 {
            n598 = local read "BD1 Frequency Out 2"() -> (w1129:u64)
            n599 = Compound Arithmetic op=AND(w1132, "Set 2", w1133) -> (w1128:bool)
            "AI2 Y Sum Set 2" <- w1131
            "AI1 X Set 2" <- w1130
          }
          frame 3 {
          }
        }
        n600 = And(x=w1092, y=w1086) -> (x .and. y?=w1093:bool)
        n601 = case shown="True" w1093 {
          tunnel: w1101 -> [_ w1152]
          tunnel: w1067 -> [_ w1151]
          tunnel: w1068 -> [_ w1150]
          tunnel: w1047 -> [_ w1149]
          tunnel: w1091 -> [_ w1148]
          tunnel: w1090 -> [_ w1147]
          tunnel: w1089 -> [_ w1146]
          tunnel: w1088 -> [_ w1145]
          tunnel: 0 ("DMA buffer timeout") -> [_ w1154]
          frame False {
          }
          frame True {
            n602 = Build Array(w1152, w1151, w1150, w1149, w1148, w1147, w1146, w1145) -> (w1153:i16[])
            n603 = for {
              tunnel: w1153 -> [w1156] mode=indexing
              tunnel: w1154 -> [w1157]
              tunnel: [w1155] -> w1143 mode=indexing
              n604 = xnode ("FIFO Write")("Element"=w1156, "Timeout"=w1157) -> ("Timed Out?"=w1155:bool)  [unwired: 1 in, 1 out]
            }
            n605 = Or Array Elements(Boolean array=w1143) -> (logical OR=w1140:bool)
            n606 = Boolean To (0,1)(Boolean=w1140) -> (0, 1=w1142:i16)
            n607 = feedback #49(u16 0) -> (w1141:u16)
            n608 = Add(x=w1142, y=w1141) -> (x+y=w1139:u16)
            "Trap AI FIFO Timeout" <- w1139
            n609 = feedback-in #49(w1139) -> ()
          }
        }
        n610 = feedback-in #47(w1070) -> ()
        n611 = feedback-in #48(w1086) -> ()
        n612 = case shown="True" w1051 {
          tunnel: w1050 -> [_ w1107]
          tunnel: [u8 0 w1104] -> w1049
          frame False {
          }
          frame True {
            n613 = Split Number(x=w1107) -> (hi(x)=w1108:u32, lo(x)=w1109:u32)
            n614 = Split Number(x=w1108) -> (lo(x)=w1110:u16)  [unwired: 1 out]
            n615 = Split Number(x=w1109) -> (hi(x)=w1111:u16, lo(x)=w1112:u16)
            n616 = Build Array "BD 1 nu Stack"(w1110, w1111, w1112) -> (w1106:u16[])
            n617 = for {
              tunnel: w1106 -> [w1119] mode=indexing
              shift-right: [w1115] -> w1104
              shift-left: u8 0 -> [w1116]
              n618 = xnode ("FIFO Method Node")("Element"=w1119, "Timeout"="Trap FIFO Set Timeout") -> ("Timed Out?"=w1118:bool)  [unwired: 1 in, 1 out]
              n619 = Boolean To (0,1)(Boolean=w1118) -> (0, 1=w1117:i16)
              n620 = To Unsigned Byte Integer(number=w1117) -> (unsigned 8bit integer=w1114:u8)
              n621 = Add(x=w1114, y=w1116) -> (x+y=w1115:u8)
            }
          }
        }
        n622 = To Unsigned Word Integer(number=w1049) -> (unsigned 16bit integer=w1048:u16)
        n623 = feedback #50(u16 0) -> (w1062:u16)
        n624 = Add(x=w1048, y=w1062) -> (x+y=w1061:u16)
        "Trap Pos FIFO Timeout" <- w1061
        n625 = feedback-in #50(w1061) -> ()
        n626 = feedback-in #51(w1085) -> ()
        n627 = feedback #51(w1085) -> (w1084:u16)
        n628 = Subtract(x=w1085, y=w1084) -> (x-y=w1083:u16)
        n629 = xnode "FPGA I/O Node"("Connector1/DIO31"=FALSE ("Connector1/DIO34")) -> ()  [unwired: 1 in, 1 out]
        n630 = Subtract(x=w1083, y=w1082) -> (x-y=w1053:u16)
        n631 = Boolean To (0,1)(Boolean="+ phase") -> (0, 1=w1078:i16)
        n632 = Multiply(x=w1078, y="Phase count adjustment") -> (x*y=w1072:i16)
        n633 = Subtract(x="ai count", y=w1053) -> (x-y=w1076:u16)
        n634 = Number To Boolean Array(number=w1053) -> (Boolean array=w1054:bool[])
        n635 = feedback #52(i16 0) -> (w1074:i16)
        n636 = Add(x=w1076, y=w1072) -> (x+y=w1075:u16)
        n637 = Subtract(x=w1074, y=w1072) -> (x-y=w1073:i16)
        "Relative phase" <- w1073
        n638 = feedback-in #52(w1073) -> ()
        n639 = Or Array Elements(Boolean array=w1054) -> (logical OR=w1052:bool)
        n640 = Boolean To (0,1)(Boolean=w1052) -> (0, 1=w1059:i16)
        n641 = To Unsigned Byte Integer(number=w1059) -> (unsigned 8bit integer=w1056:u8)
        n642 = feedback #53(u8 0) -> (w1057:u8)
        n643 = Add(x=w1056, y=w1057) -> (x+y=w1055:u8)
        "AI Late Counter" <- w1055
        n644 = feedback-in #53(w1055) -> ()
      }
    }
  }
  n645 = node-c288(w8) -> ()
  n646 = while "APD 3 Counter" {
    tunnel: w2 -> [_]
    stop <- FALSE stop-if-true
    n647 = flat-sequence {
      frame #0 {
        n648 = xnode "FPGA I/O Method Node"("FPGA I/O In"=refnum<k21> "Connector0/DIO2" ("APD 2 DO"), "Timeout"=-1) -> ()  [unwired: 2 out]
      }
      frame #1 {
        n649 = local read "APD3 int gate"() -> (w1161:bool)
        n650 = case shown="True" w1161 {
          frame False {
          }
          frame True {
            n651 = local read "APD3 out state"() -> (w1162:bool)
            n652 = case shown="True" w1162 {
              frame False {
                n653 = local read "APD 3 Counts 0"() -> (w1164:u32)
                n654 = Increment(x=w1164) -> (x+1=→"APD 3 Counts 0":u32)
              }
              frame True {
                n655 = local read "APD 3 Counts 1"() -> (w1166:u32)
                n656 = Increment(x=w1166) -> (x+1=→"APD 3 Counts 1":u32)
              }
            }
          }
        }
      }
    }
  }
  n657 = while "APD 3 Gating" {
    shift-right: [w1170] -> _
    shift-left: w2 -> [w1175]
    shift-right: [w1169] -> _
    shift-left: w6 -> [w1167]
    stop <- FALSE stop-if-true
    n658 = flat-sequence {
      tunnel: w1175 -> [w1178]
      tunnel: [w1179] -> w1173
      tunnel: [w1178] -> w1171
      tunnel: [w1177] -> w1168
      tunnel: w1167 -> [w1177]
      tunnel: [w1182] -> w1174
      tunnel: w1173 -> [w1182]
      tunnel: [w1181] -> w1172
      tunnel: w1171 -> [w1181]
      tunnel: w1168 -> [w1180]
      tunnel: [w1203] -> w1170
      tunnel: w1174 -> [w1214]
      tunnel: w1172 -> [w1211]
      tunnel: [w1183] -> w1169
      frame #0 {
        n659 = call "Loop Timer15"("Count(Ticks)"=w1178) -> ("Tick Count(Ticks)"=w1179:u16)
      }
      frame #1 {
        # "Signal maybe then sent through \na transistor before APD"
        n660 = xnode "FPGA I/O Node"("Connector0/DIO12"=w1180, "Connector0/DIO13"=w1180, "Connector0/DIO14"=w1180, "Connector0/DIO15"=w1180) -> ()  [unwired: 4 in, 4 out]
        "APD3 int gate" <- w1180
      }
      frame #2 {
        n661 = local read "APD Gate OFF Count"() -> (w1188:u16)
        n662 = local read "APD Gate ON Count"() -> (w1189:u16)
        n663 = feedback #54(TRUE) -> (w1208:bool)
        n664 = feedback-in #55(w1214) -> ()
        n665 = feedback #55(w1214) -> (w1213:u16)
        n666 = Not(x=w1208) -> (.not. x?=w1206:bool)
        n667 = feedback-in #54(w1206) -> ()
        n668 = Subtract(x=w1214, y=w1213) -> (x-y=w1212:u16)
        n669 = Select(t=w1189, s=w1206, f=w1188) -> (s? t:f=w1210:u16)
        n670 = Subtract(x=w1212, y=w1211) -> (x-y=w1191:u16)
        n671 = Subtract(x=w1210, y=w1191) -> (x-y=w1202:u16)
        n672 = Number To Boolean Array(number=w1191) -> (Boolean array=w1192:bool[])
        n673 = Or Array Elements(Boolean array=w1192) -> (logical OR=w1190:bool)
        n674 = Boolean To (0,1)(Boolean=w1190) -> (0, 1=w1197:i16)
        n675 = Boolean To (0,1)(Boolean="+ phase (APD 3 Gate)") -> (0, 1=w1200:i16)
        n676 = To Unsigned Byte Integer(number=w1197) -> (unsigned 8bit integer=w1194:u8)
        n677 = Multiply(x=w1200, y="Phase count adjustment (APD 3 Gate)") -> (x*y=w1198:i16)
        n678 = feedback #56(u8 0) -> (w1195:u8)
        n679 = Add(x=w1194, y=w1195) -> (x+y=w1193:u8)
        "APD 3 Gate Late Counter" <- w1193
        n680 = feedback-in #56(w1193) -> ()
        n681 = Add(x=w1202, y=w1198) -> (x+y=w1203:u16)
        n682 = feedback #57(i16 0) -> (w1205:i16)
        n683 = Subtract(x=w1205, y=w1198) -> (x-y=w1204:i16)
        "APD 3 Gate Relative Phase" <- w1204
        n684 = feedback-in #57(w1204) -> ()
        n685 = local read "APD Gate Operating Mode"() -> (w1187:u8)
        n686 = case shown="2" w1187 {
          tunnel: [TRUE FALSE w1217] -> w1184
          tunnel: w1208 -> [_ _ w1217]
          frame 0, Default {
          }
          frame 1 {
          }
          frame 2 {
          }
        }
        n687 = local read "Invert APD Gate"() -> (w1186:bool)
        n688 = Not(x=w1184) -> (.not. x?=w1185:bool)
        n689 = Select(t=w1185, s=w1186, f=w1184) -> (s? t:f=w1183:bool)
      }
    }
  }
  n690 = while "633 nm red  fluorescent laser interlacing (DO to IA 633 nm AOM ME amp)." {
    shift-right: [w1221] -> _
    shift-left: w2 -> [w1226]
    shift-right: [w1220] -> _
    shift-left: w3 -> [w1218]
    stop <- FALSE stop-if-true
    n691 = flat-sequence {
      tunnel: w1226 -> [w1229]
      tunnel: [w1230] -> w1224
      tunnel: [w1229] -> w1222
      tunnel: [w1228] -> w1219
      tunnel: w1218 -> [w1228]
      tunnel: [w1233] -> w1225
      tunnel: w1224 -> [w1233]
      tunnel: [w1232] -> w1223
      tunnel: w1222 -> [w1232]
      tunnel: w1219 -> [w1231]
      tunnel: [w1242] -> w1221
      tunnel: w1225 -> [w1262]
      tunnel: w1223 -> [w1259]
      tunnel: [w1251] -> w1220
      frame #0 {
        n692 = call "Loop Timer11"("Count(Ticks)"=w1229) -> ("Tick Count(Ticks)"=w1230:u16)
      }
      frame #1 {
        # "Then to PRL 440 amp"
        n693 = xnode "FPGA I/O Node"("Connector1/DIO32"=w1231) -> ()  [unwired: 1 in, 1 out]
      }
      frame #2 {
        n694 = feedback-in #58(w1262) -> ()
        n695 = feedback #58(w1262) -> (w1261:u16)
        n696 = Subtract(x=w1262, y=w1261) -> (x-y=w1260:u16)
        n697 = Subtract(x=w1260, y=w1259) -> (x-y=w1235:u16)
        n698 = Number To Boolean Array(number=w1235) -> (Boolean array=w1236:bool[])
        n699 = Or Array Elements(Boolean array=w1236) -> (logical OR=w1234:bool)
        n700 = Boolean To (0,1)(Boolean="+ phase (RI)") -> (0, 1=w1247:i16)
        n701 = Multiply(x=w1247, y="Phase count adjustment (RI)") -> (x*y=w1244:i16)
        n702 = Boolean To (0,1)(Boolean=w1234) -> (0, 1=w1241:i16)
        n703 = To Unsigned Byte Integer(number=w1241) -> (unsigned 8bit integer=w1238:u8)
        n704 = feedback #59(i16 0) -> (w1245:i16)
        n705 = feedback #60(u8 0) -> (w1239:u8)
        n706 = Add(x=w1238, y=w1239) -> (x+y=w1237:u8)
        "RI Late Counter" <- w1237
        n707 = feedback-in #60(w1237) -> ()
        n708 = Subtract(x=w1245, y=w1244) -> (x-y=w1243:i16)
        "RI Relative phase" <- w1243
        n709 = feedback-in #59(w1243) -> ()
        n710 = feedback #61(TRUE) -> (w1254:bool)
        n711 = case shown="2" "Red Laser Operating Mode" {
          tunnel: [TRUE FALSE w1268] -> w1251
          tunnel: w1254 -> [_ _ w1265]
          frame 0, Default {
          }
          frame 1 {
          }
          frame 2 {
            n712 = Not(x=w1265) -> (.not. x?=w1267:bool)
            n713 = Select(t=w1267, s="Invert RI", f=w1265) -> (s? t:f=w1268:bool)
          }
        }
        n714 = Not(x=w1254) -> (.not. x?=w1250:bool)
        n715 = Select(t="Red interlace ON count", s=w1250, f="Red interlace OFF count") -> (s? t:f=w1256:u16)
        n716 = Subtract(x=w1256, y=w1235) -> (x-y=w1248:u16)
        n717 = Add(x=w1248, y=w1244) -> (x+y=w1242:u16)
        n718 = feedback-in #61(w1250) -> ()
      }
    }
  }
  n719 = while "473 nm blue  fluorescent laser interlacing (DO to blue laser digital control input)." {
    shift-right: [w1272] -> _
    shift-left: w2 -> [w1277]
    shift-right: [w1271] -> _
    shift-left: w3 -> [w1269]
    stop <- FALSE stop-if-true
    n720 = flat-sequence {
      tunnel: w1277 -> [w1280]
      tunnel: [w1281] -> w1275
      tunnel: [w1280] -> w1273
      tunnel: [w1279] -> w1270
      tunnel: w1269 -> [w1279]
      tunnel: [w1284] -> w1276
      tunnel: w1275 -> [w1284]
      tunnel: [w1283] -> w1274
      tunnel: w1273 -> [w1283]
      tunnel: w1270 -> [w1282]
      tunnel: [w1293] -> w1272
      tunnel: w1276 -> [w1313]
      tunnel: w1274 -> [w1310]
      tunnel: [w1302] -> w1271
      frame #0 {
        n721 = call "Loop Timer14"("Count(Ticks)"=w1280) -> ("Tick Count(Ticks)"=w1281:u16)
      }
      frame #1 {
        n722 = xnode "FPGA I/O Node"("Connector1/DIO28"=w1282) -> ()  [unwired: 1 in, 1 out]
      }
      frame #2 {
        n723 = feedback-in #62(w1313) -> ()
        n724 = feedback #62(w1313) -> (w1312:u16)
        n725 = Subtract(x=w1313, y=w1312) -> (x-y=w1311:u16)
        n726 = Subtract(x=w1311, y=w1310) -> (x-y=w1286:u16)
        n727 = Number To Boolean Array(number=w1286) -> (Boolean array=w1287:bool[])
        n728 = Or Array Elements(Boolean array=w1287) -> (logical OR=w1285:bool)
        n729 = Boolean To (0,1)(Boolean="+ phase (BI D)") -> (0, 1=w1298:i16)
        n730 = Multiply(x=w1298, y="Phase count adjustment (BI D)") -> (x*y=w1295:i16)
        n731 = Boolean To (0,1)(Boolean=w1285) -> (0, 1=w1292:i16)
        n732 = To Unsigned Byte Integer(number=w1292) -> (unsigned 8bit integer=w1289:u8)
        n733 = feedback #63(i16 0) -> (w1296:i16)
        n734 = feedback #64(u8 0) -> (w1290:u8)
        n735 = Add(x=w1289, y=w1290) -> (x+y=w1288:u8)
        "Blue Late Counter (D)" <- w1288
        n736 = feedback-in #64(w1288) -> ()
        n737 = Subtract(x=w1296, y=w1295) -> (x-y=w1294:i16)
        "BI Relative phase (D)" <- w1294
        n738 = feedback-in #63(w1294) -> ()
        n739 = feedback #65(TRUE) -> (w1305:bool)
        n740 = case shown="2" "Blue Laser Operating Mode (D)" {
          tunnel: [TRUE FALSE w1319] -> w1302
          tunnel: w1305 -> [_ _ w1316]
          frame 0, Default {
          }
          frame 1 {
          }
          frame 2 {
            n741 = Not(x=w1316) -> (.not. x?=w1318:bool)
            n742 = Select(t=w1318, s="Invert BI (D)", f=w1316) -> (s? t:f=w1319:bool)
          }
        }
        n743 = Not(x=w1305) -> (.not. x?=w1301:bool)
        n744 = Select(t="Blue interlace ON count (D)", s=w1301, f="Blue interlace OFF count (D)") -> (s? t:f=w1307:u16)
        n745 = Subtract(x=w1307, y=w1286) -> (x-y=w1299:u16)
        n746 = Add(x=w1299, y=w1295) -> (x+y=w1293:u16)
        n747 = feedback-in #65(w1301) -> ()
      }
    }
  }
  n748 = while "Blue fluorescent laser interlacing (AO control direct to laser)." {
    shift-right: [w1325] -> _
    shift-left: w2 -> [w1328]
    shift-right: [w1322] -> _
    shift-left: i16 0 -> [w1320]
    stop <- FALSE stop-if-true
    n749 = flat-sequence {
      tunnel: w1328 -> [w1331]
      tunnel: [w1332] -> w1327
      tunnel: [w1331] -> w1326
      tunnel: [w1330] -> w1321
      tunnel: w1320 -> [w1330]
      tunnel: [w1335] -> w1324
      tunnel: w1327 -> [w1335]
      tunnel: [w1334] -> w1323
      tunnel: w1326 -> [w1334]
      tunnel: w1321 -> [w1333]
      tunnel: [w1345] -> w1325
      tunnel: [w1361] -> w1322
      tunnel: w1324 -> [w1373]
      tunnel: w1323 -> [w1370]
      frame #0 {
        n750 = call "Loop Timer13"("Count(Ticks)"=w1331) -> ("Tick Count(Ticks)"=w1332:u16)
      }
      frame #1 {
        n751 = xnode "FPGA I/O Node"("Connector0/AO3"=w1333) -> ()  [unwired: 1 in, 1 out]
      }
      frame #2 {
        n752 = Subtract(x="Blue OFF count (AO)", y="Blue current ON count adj (AO)") -> (x-y=w1354:u16)
        n753 = feedback-in #66(w1373) -> ()
        n754 = feedback #66(w1373) -> (w1372:u16)
        n755 = Add(x="Blue current ON count adj (AO)", y="Blue ON count (AO)") -> (x+y=w1355:u16)
        n756 = Subtract(x=w1373, y=w1372) -> (x-y=w1371:u16)
        n757 = Subtract(x=w1371, y=w1370) -> (x-y=w1338:u16)
        n758 = Number To Boolean Array(number=w1338) -> (Boolean array=w1339:bool[])
        n759 = Boolean To (0,1)(Boolean="+ phase (BI AO)") -> (0, 1=w1351:i16)
        n760 = Or Array Elements(Boolean array=w1339) -> (logical OR=w1337:bool)
        n761 = Boolean To (0,1)(Boolean=w1337) -> (0, 1=w1344:i16)
        n762 = Multiply(x=w1351, y="Phase count adjustment (BI AO)") -> (x*y=w1347:i16)
        n763 = To Unsigned Byte Integer(number=w1344) -> (unsigned 8bit integer=w1340:u8)
        n764 = feedback #67(u8 0) -> (w1342:u8)
        n765 = Add(x=w1340, y=w1342) -> (x+y=w1341:u8)
        "BI Late Counter (AO)" <- w1341
        n766 = feedback-in #67(w1341) -> ()
        n767 = feedback #68(i16 0) -> (w1348:i16)
        n768 = Subtract(x=w1348, y=w1347) -> (x-y=w1346:i16)
        "BI Relative phase (AO)" <- w1346
        n769 = feedback-in #68(w1346) -> ()
        n770 = feedback #69(TRUE) -> (w1365:bool)
        n771 = case shown="2" "BI Operating Mode (AO)" {
          tunnel: [TRUE FALSE w1389] -> w1356
          tunnel: w1365 -> [_ _ w1386]
          frame 0, Default {
          }
          frame 1 {
          }
          frame 2 {
            n772 = Not(x=w1386) -> (.not. x?=w1388:bool)
            n773 = Select(t=w1388, s="Invert BI (AO)", f=w1386) -> (s? t:f=w1389:bool)
          }
        }
        n774 = And(x=w1356, y="Blue FB On/Off") -> (x .and. y?=w1357:bool)
        n775 = case shown="True" w1357 {
          tunnel: "BI Current Out" -> [w1374 _]
          tunnel: [w1374 w1376] -> w1360
          frame False {
          }
          frame True {
            n776 = local read "Blue Intensity"() -> (w1375:i16)
            n777 = Bundle("P5"="P5", "I5"="I5", "D5"="D5") -> (w1377:cluster{"P5":i16, "I5":i16, "D5":i16})  [unwired: 1 in]
            n778 = call "Slower PID.vi"("process variable"=w1375, "reset?"="Blue FB Reset", "setpoint"="Blue FB Setpoint", "PID gains (x 2^8)"=w1377, "output range"=cluster{"output high":i16, "output low":i16} {"output high"=32767, "output low"=0} ("Green FB output range")) -> ("output"=w1376:i16)  [unwired: 10 out]
          }
        }
        n779 = Not(x=w1365) -> (.not. x?=w1362:bool)
        n780 = Select(t=w1355, s=w1362, f=w1354) -> (s? t:f=w1367:u16)
        n781 = Subtract(x=w1367, y=w1338) -> (x-y=w1349:u16)
        n782 = Add(x=w1349, y=w1347) -> (x+y=w1345:u16)
        n783 = feedback-in #69(w1362) -> ()
        n784 = Boolean To (0,1)(Boolean=w1356) -> (0, 1=w1336:i16)
        n785 = Multiply(x=w1336, y=w1360) -> (x*y=w1361:i16)
      }
    }
  }
